vi "Server Main Simplicity.vi"() -> ()   [LabVIEW 2015]
doc: "Use this template to create an application that executes until you click the Stop button. Unlike the Single Loop Application VI that uses polling, this VI uses the Event structure."
uses:
  Type/_Server Command.ctl
  Type/_Run State.ctl
  Type/_Log Command.ctl
  <vilib>/registry/registry.llb/Registry SAM.ctl
  Type/_RT Command.ctl
  Configuration/AcquisitionState.ctl
  Type/_RT Instrument State.ctl
  Type/_Source Type.ctl
  <vilib>/Utility/config.llb/Read Key (Path).vi
  <vilib>/Utility/config.llb/Write Key (Path).vi
  <vilib>/Utility/config.llb/Read Key (String).vi
  <vilib>/Utility/config.llb/Write Key (String).vi
  Configuration/_Global Configuration.vi
  <vilib>/registry/registry.llb/Write Registry Value Simple STR.vi
  <vilib>/Utility/config.llb/Read Key (Boolean).vi
  <vilib>/Utility/config.llb/Read Key (I32).vi
  _Server Global.vi
  <vilib>/Utility/config.llb/NI_LVConfig.lvlib
panel:
  out "MS Status":string="Simulation (State = Ready)"
  in  "MSStatusWindow":bool
  in  "MSShutDown":bool
  in  "MSStart":bool
  out "S2Type":i8(ring)=2 items=["None", "ESI", "APCI", "APPI", "MicroSpray"]
  out "S1Type":i8(ring)=1 items=["None", "ESI", "APCI", "APPI", "MicroSpray"]
  out "S2Temp":sgl caption="Data Queue"
  out "S1Temp":sgl=125.0 caption="Data Queue"
  out "HSIDTemp":sgl=300.0 caption="Data Queue"
  in  "Negative":bool
  in  "Positive":bool
  out "MS Ready":u16(ring)=2
  in  "ContactClosures":bool
  out "Corona Discharge:":sgl format="%.1f"
  out "ElectroSpray V2:":sgl
  out "ElectroSpray V1:":sgl
  in  "GetStatus":bool
  out "Heating Gas 2:":sgl
  out "Heating Gas 1:":sgl
  out "Nebulizer Gas 1:":sgl
  out "Nebulizer Gas 2:":sgl
  out "Collision Pressure:":sgl format="%.1f"
  out "Dry Gas:":sgl
  out "Exhaust:":sgl
  out "Pump Speed:":sgl
  out "Exhaust OK":bool
  out "CurGas OK":bool
  out "Pump OK":bool
  out "Interlock OK":bool
  out "Vac. Pressure:":sgl format="%.2e"
  out "Scans":i32 caption="Data Queue"
  out "Engine Error":errorcluster
  out "Connected":bool
  out "Error":string
  out "Data":string
  out "Ready":bool=TRUE
  in  "Command":T1=enum."Get Status"
  in  "Message":string="<Method>\n  1\t0\t0\n  <Experiment>\n    1\t0\t0\t200\t0\t100\t1\t0\n    <MassRange>\n      200.000000\t400\t0.100000\t2000\t0.1\t0\n      <ParamTable/>\n    </MassRange>\n  </Experiment>\n</Method>"
  out "Data Queue":i32
  out "Busy":bool
  out "Locked":bool
  # "Mass Calibration & Resolution"
  # "Source"
  # "1"
  # "2"
  # "HSID"
  # "Simplicity Server V6.5 R&D"
  # "Source 1"
  # "Common Interface"
  # "Source 2"
  # "Other Status"
  # "Torr"
  # "Interlocks:"
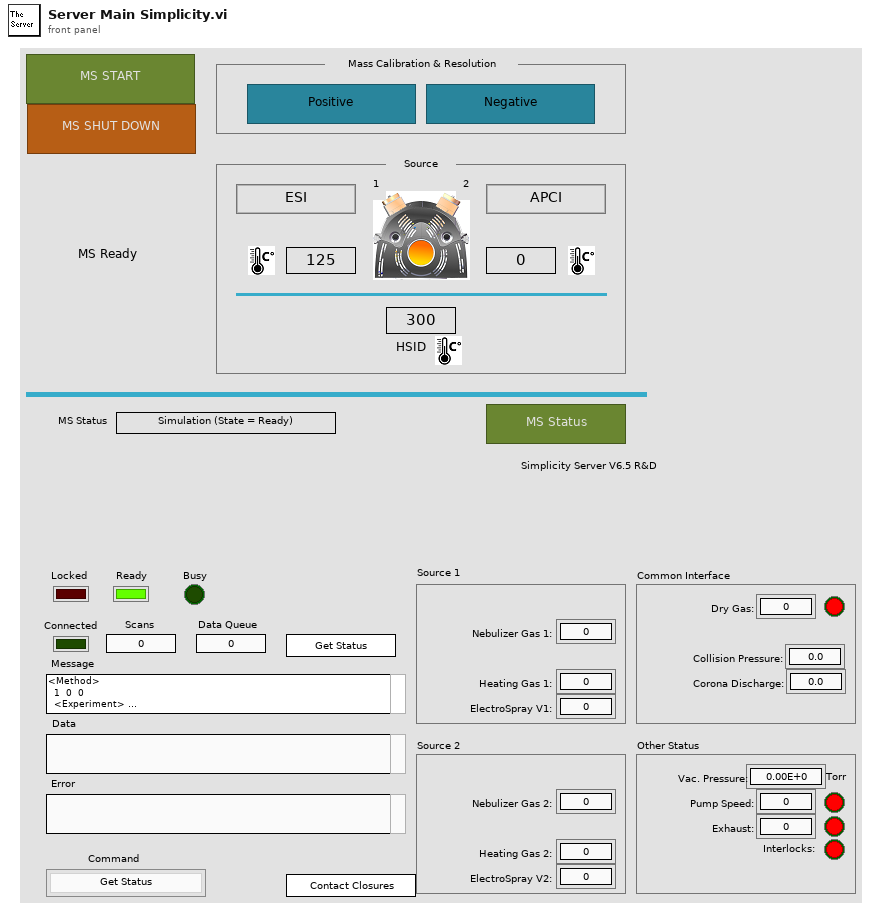
[diagram p1: front panel]
types:
  T1 = typedef "_Server Command.ctl" = enum16{"Hide Server", "Show Server", "Close Server", "Start Run", "Start Actual Run", "Stop Run", "Runtime Update", "Get Data", "Get Status", "Get Table", "Set Table", "Get Configuration", "Reserved", "Get Memory Map", "Read ADC", "Set Oscillator", "Reboot", "Backup Firmware", "Update Firmware", "Auxiliary Update", "System Status", "Start System", "Shutdown System", "Start LC Equilibration", "Get LC Status", "Get LC Configuration", "Get LC Method Contents", "Rinse Autosampler", "Pump OnOff", "Oven OnOff", "Get LC Error", "Clear LC Error", "Set LC Input Logic", "Set LC Hold Logic", "Lock Server", "Get Current Method", "Get Real Time Data", "Connect LC", "Disconnect LC"}
  T2 = typedef "_Run State.ctl" = enum16{"Init", "Update", "Start", "End", "Error"}
  T3 = typedef "_Log Command.ctl" = enum16{"No Command", "Open", "Read", "Write", "Close", "Check Size"}
  T4 = typedef "AcquisitionState.ctl" = enum16{"Ready", "Busy", "Waiting"}
  T5 = enum32{"Invalid", "Standard", "Closed", "Hidden", "Minimized", "Maximized"}
  T6 = typedef "_RT Command.ctl" = enum16{"xml Start Run", "xml Start Actual Run", "xml Stop Run", "xml Runtime Update", "xml Get Status", "xml Get Table", "xml Set Table", "xml Get Configuration", "xml System Status", "xml Set LC Input Logic", "xml Get Data", "xml Get Info", "Start", "StartActualRun", "Stop", "Runtime Update", "Get Data", "Get Info", "Get Status", "Get Param", "Get Config", "Get Table", "Read ADC", "Set Oscillator", "Update Config", "Update Table", "Set All Pol", "Set Pol and DC", "Set Max Mass", "Toggle RP", "Toggle EL", "Set PIC", "Initialize Turbo", "Send Turbo Comm", "Close Turbo", "P1", "P2", "P3", "Send Serial", "Set LC Out", "Get LC In", "Read VAC", "Test Table", "Toggle Power", "Get Startup", "Set Startup", "Get ADC Table", "Set ADC Table", "Get Brief Status", "Get Detail Status", "Auxiliary Update", "Set CC Logics", "Set CC Input Logics", "Ignore Error", "invalid"}
  T7 = typedef "Registry SAM.ctl" = enum32{"KEY_QUERY_VALUE", "KEY_SET_VALUE", "KEY_CREATE_SUB_KEY", "KEY_ENUMERATE_SUB_KEYS", "KEY_NOTIFY", "KEY_CREATE_LINK", "KEY_READ", "KEY_WRITE", "KEY_ALL_ACCESS", "KEY_READ | KEY_WRITE"}
  T8 = enum8{"Enabled", "Disabled", "Disabled and Grayed Out"}
  T9 = enum32{"Bad", "Idle", "Run top level", "Running"}
  T10 = typedef "NI_LVConfig.lvlib/Config Data RefNum.ctl" = refnum<k1>
  T11 = typedef "Registry refnum.ctl" = refnum<k1>
  T12 = typedef "_RT Instrument State.ctl" = enum16{"Initializing", "Mass Spectrometer is Off", "Starting Up", "Turning Power Off", "Going to Standby", "Roughing Pump Ready", "Turning Turbo Off", "Turbo Startup", "Turbopump Ready", "Checking Vacuum", "Going to Ready", "Ready", "Running", "Source Standby", "Lost Communication", "Shutting Down", "Fault", "24V Standby", "Go to 24V Standby", "Turbopump Ready-Waiting"}
  T13 = cluster{"InstrState":T12, "RT Ready":bool, "LockServer":bool, "LastGetStatusTime":u32}
  T14 = typedef "_XML Lens.ctl" = cluster{"Value":dbl, "ChID":u8}
  T15 = typedef "_RT Instrument 2.ctl" = cluster{"Table":T16[], "Instrument":string[]}
  T16 = typedef "_RT Configuration 2.ctl" = cluster{"Name":string, "Ch#":u8, "Min":dbl, "Max":dbl, "Def+":dbl, "Def-":dbl, "Offset":dbl, "Slope":dbl, "Type":u8, "Description":string, "SettleT":dbl}
  T17 = cluster{"value":string, string, path, "Source":enum32{"RT Target", "Folder"}}
  T18 = typedef "_Source Type.ctl" = i8
  T19 = typedef "_Brief Status.ctl" = cluster{"Source 1 Type: ":T18, "Nebulizer Gas 1:":sgl, "Probe Temp 1: ":sgl, "Heating Gas 1:":sgl, "Source 2 Type:  ":T18, "Nebulizer Gas 2:":sgl, "Probe Temp 2: ":sgl, "Heating Gas 2:":sgl, "Dry Gas:":sgl, "HSID Temp:  ":sgl, "Collision Gas:":sgl, "Vac. Pressure: ":sgl, "Pump Speed:":sgl, "Exhaust:":sgl, "Interlock OK":bool, "CurGas OK":bool, "Pump OK":bool, "Exhaust OK":bool, "Event":string, "Corona Discharge:":sgl, "Source 1 Voltage:":sgl, "Source 2 Voltage:":sgl}
  T20 = enum16{"Left Button", "Center Button", "Right Button", "Window Close"}
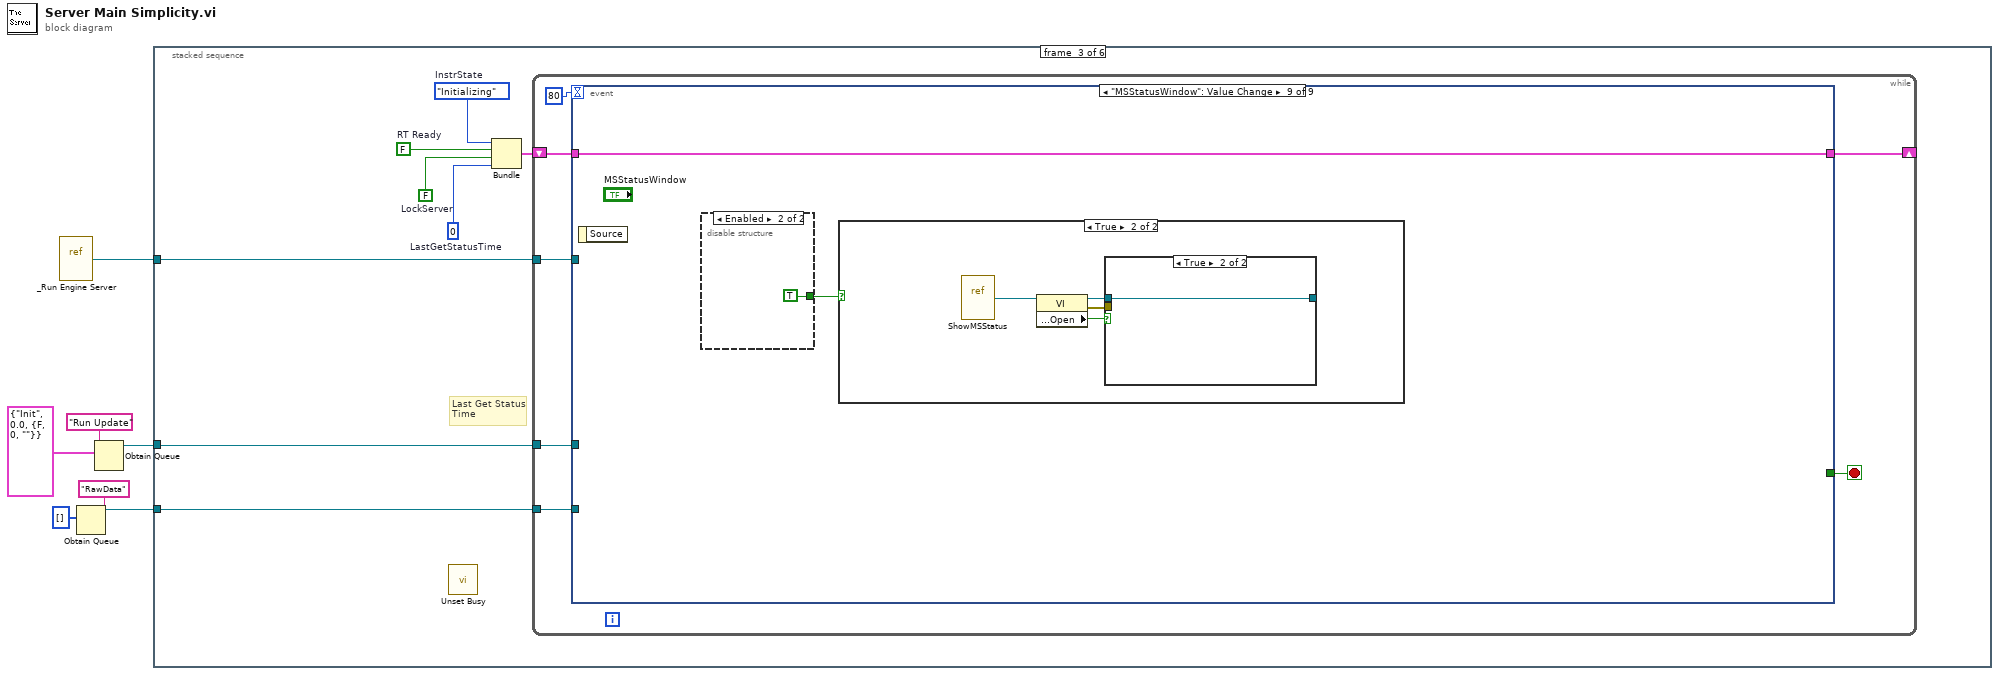
[diagram p0: block diagram]
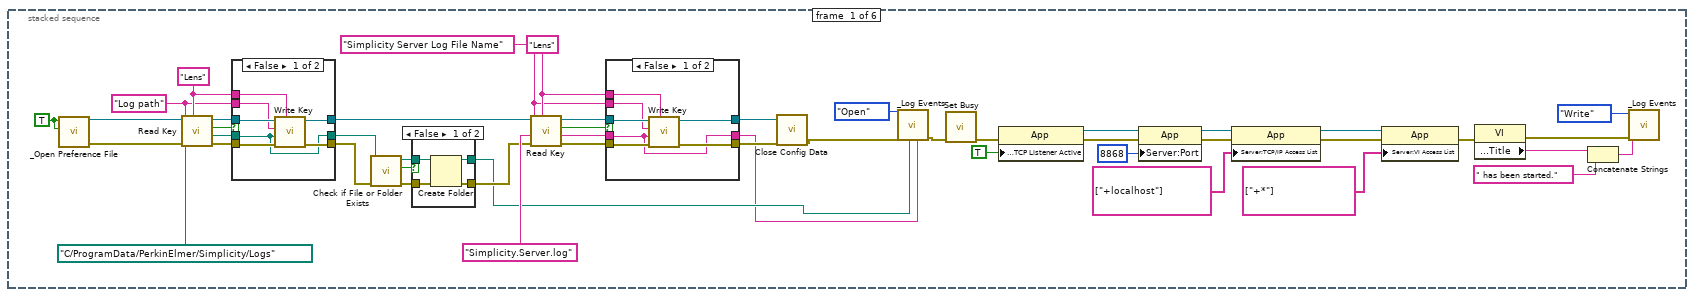
[diagram p2: hidden frame]
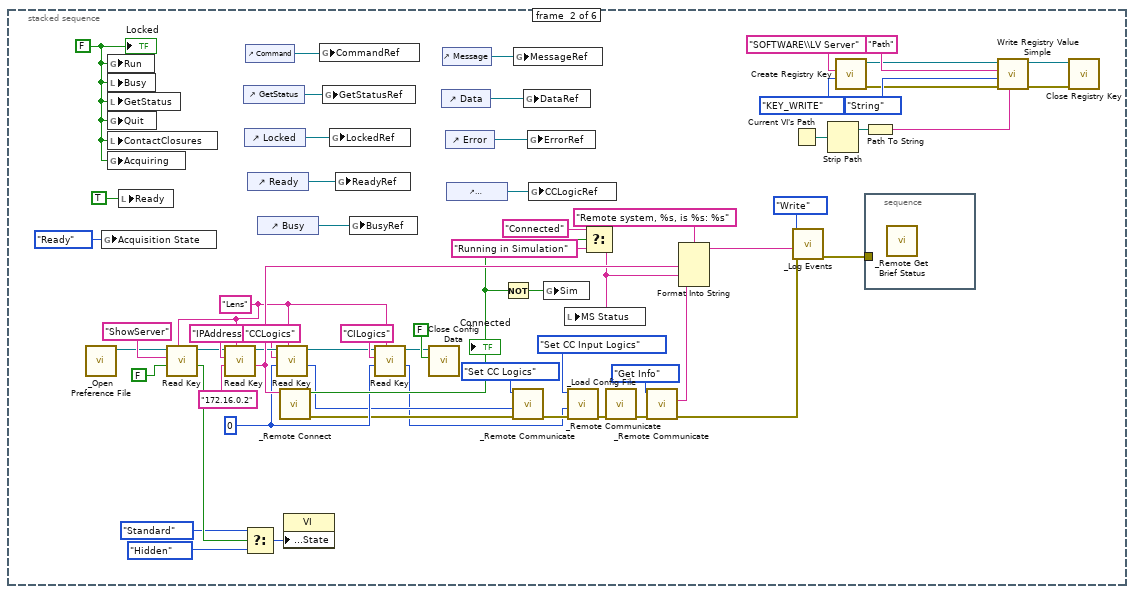
[diagram p6: hidden frame]
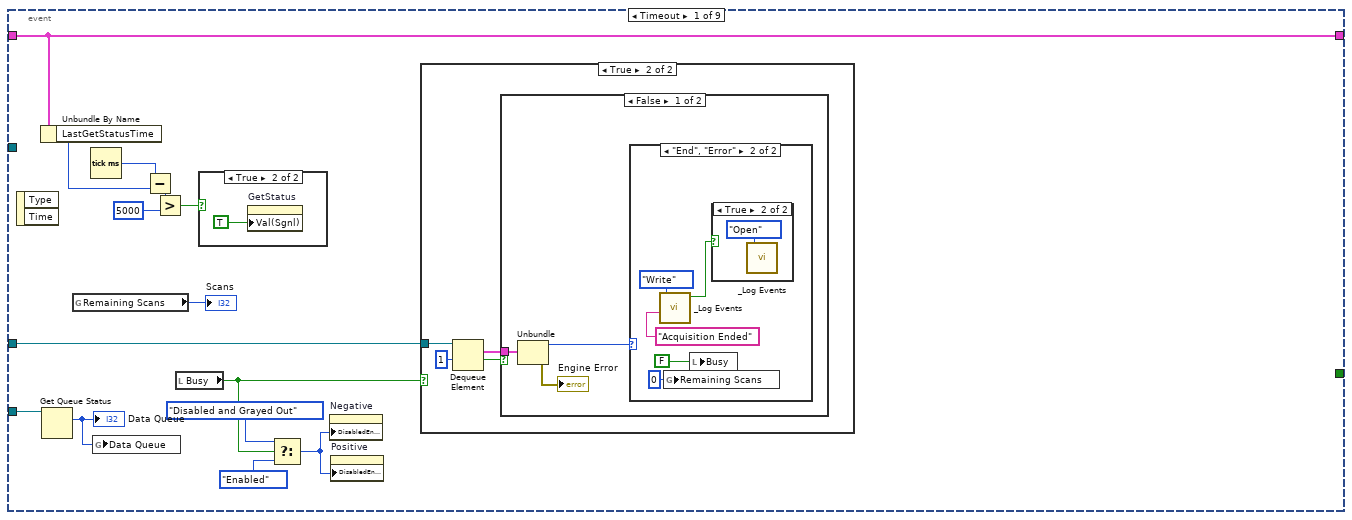
[diagram p7: hidden frame]
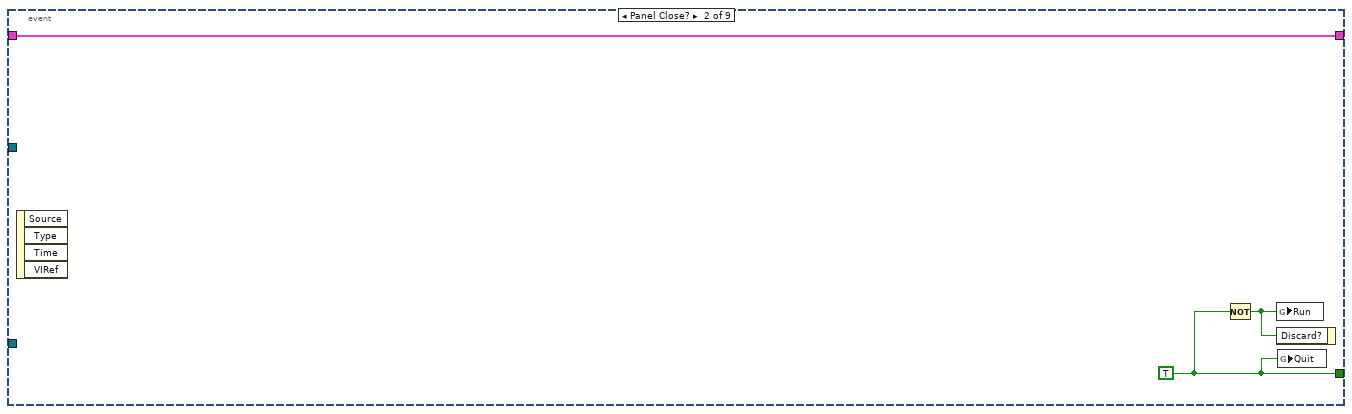
[diagram p13: hidden frame]
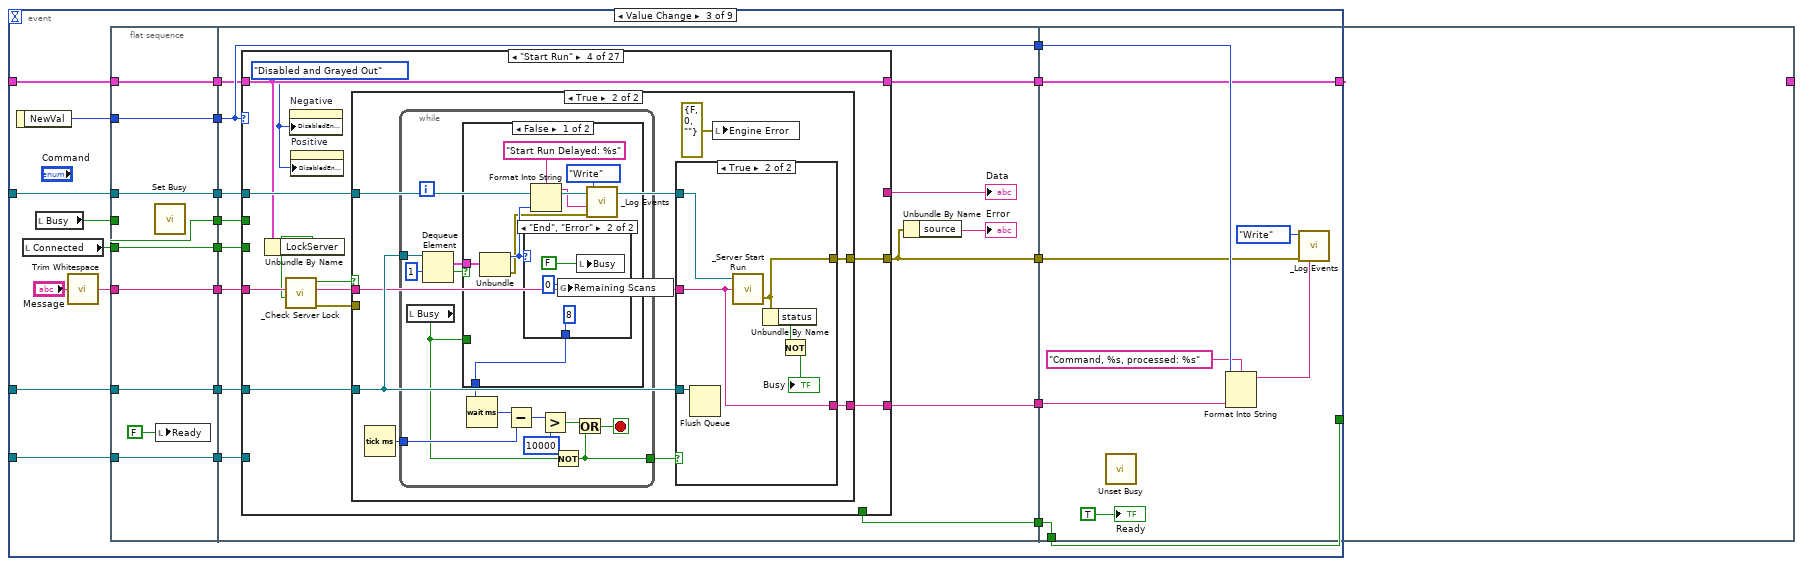
[diagram p14: hidden frame]
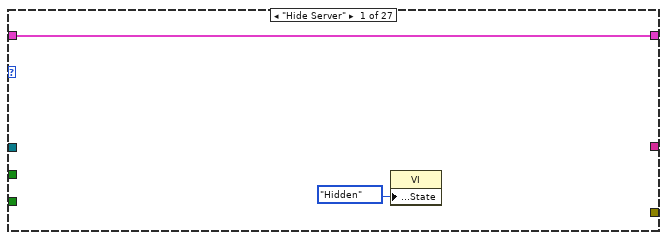
[diagram p15: hidden frame]
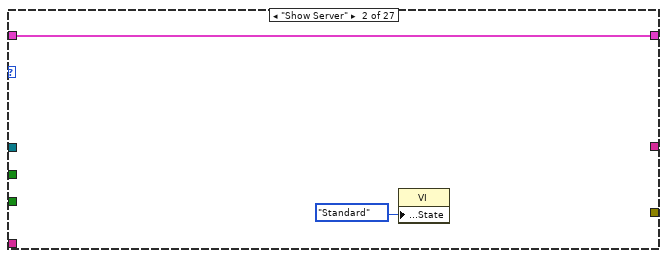
[diagram p16: hidden frame]
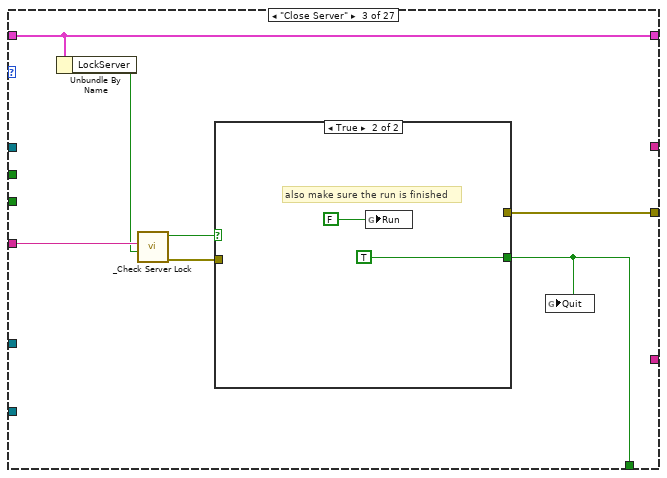
[diagram p17: hidden frame]
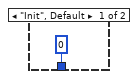
[diagram p20: hidden frame]
diagram:
  n1 = vi-ref "_Run Engine Server.vi"() -> (w5:refnum<vi>)
  n2 = Obtain Queue(name (unnamed)="RawData", element data type=i32[] []) -> (queue out=w1:refnum<queue>)  [unwired: 3 in, 2 out]
  n3 = Obtain Queue(name (unnamed)="Run Update", element data type=cluster{T2, dbl, "error out":errorcluster} {enum."Init", 0.0, "error out"={"status"=FALSE, "code"=0, "source"=""}}) -> (queue out=w4:refnum<queue>)  [unwired: 3 in, 2 out]
  n4 = stacked-sequence {
    tunnel: w4 -> [_ _ w151 _ _ _]
    tunnel: w5 -> [_ _ w150 _ _ _]
    tunnel: w1 -> [_ _ w144 _ _ _]
    frame #0 {
      w21 = "Simplicity Server Log File Name" ("key")
      w22 = "Lens" ("section")
      w27 = "Log path" ("key")
      w28 = "Lens" ("section")
      w36 = TRUE ("Server")
      n5 = call "_Open Preference File.vi"("Initialize"=w36, "Server"=w36) -> ("error"=w17:errorcluster, "refnum"=w18:T10)  [unwired: 1 in, 3 out]
      n6 = call-poly <vilib>:"Read Key.vi"("section"=w28, "error in (no error)"=w17, "default value"=path "C:/ProgramData/PerkinElmer/Simplicity/Logs", "key"=w27, "refnum"=w18) -> ("error out"=w33:errorcluster, "value"=w31:path, "found?"=w32:bool, "refnum out"=w30:T10)  [unwired: 3 in]
      n7 = case shown="False" w32 {
        tunnel: w33 -> [w78 w81]
        tunnel: w31 -> [w72 w79]
        tunnel: w30 -> [w76 w80]
        tunnel: [w77 w81] -> w11
        tunnel: [w75 w80] -> w29
        tunnel: [w72 w79] -> w12
        tunnel: w28 -> [w74 _]
        tunnel: w27 -> [w73 _]
        frame False {
          n8 = call-poly <vilib>:"Write Key.vi"("section"=w74, "error in (no error)"=w78, "value"=w72, "key"=w73, "refnum"=w76) -> ("error out"=w77:errorcluster, "refnum out"=w75:T10)  [unwired: 4 in, 1 out]
        }
        frame True {
        }
      }
      n9 = call <vilib>:"Check if File or Folder Exists.vi"("error in (no error)"=w11, "path"=w12) -> ("error out"=w15:errorcluster, "file or folder exists?"=w13:bool, "dup path"=w14:path)  [unwired: 7 in]
      n10 = case shown="False" w13 {
        tunnel: w15 -> [w59 w60]
        tunnel: w14 -> [w58 w61]
        tunnel: [w57 w61] -> w9
        tunnel: [w56 w60] -> w10
        frame False {
          n11 = Create Folder(path (use dialog)=w58, error in=w59) -> (created path=w57:path, error out=w56:errorcluster)  [unwired: 1 in, 1 out]
        }
        frame True {
        }
      }
      n12 = call-poly <vilib>:"Read Key.vi"("section"=w22, "error in (no error)"=w10, "default value"="Simplicity.Server.log", "key"=w21, "refnum"=w29) -> ("error out"=w23:errorcluster, "value"=w24:string, "found?"=w25:bool, "refnum out"=w26:T10)  [unwired: 3 in]
      n13 = case shown="False" w25 {
        tunnel: w23 -> [w68 w71]
        tunnel: w24 -> [w62 w69]
        tunnel: w26 -> [w66 w70]
        tunnel: [w67 w71] -> w19
        tunnel: [w65 w70] -> w20
        tunnel: [w62 w69] -> w8
        tunnel: w22 -> [w64 _]
        tunnel: w21 -> [w63 _]
        frame False {
          n14 = call-poly <vilib>:"Write Key.vi"("section"=w64, "error in (no error)"=w68, "value"=w62, "key"=w63, "refnum"=w66) -> ("error out"=w67:errorcluster, "refnum out"=w65:T10)  [unwired: 4 in, 1 out]
        }
        frame True {
        }
      }
      n15 = call <vilib>:"Close Config Data.vi"("error in (no error)"=w19, "refnum"=w20) -> ("error out"=w16:errorcluster)  [unwired: 1 in, 8 out]
      n16 = call "_Log Events.vi"("File Name"=w8, "Log Path"=w9, "error in (no error)"=w16, "Log Command"=_Log_Command."Open" ("File Command")) -> ("error out"=w37:errorcluster)  [unwired: 4 in, 1 out]
      n17 = call <vilib>:"Set Busy.vi"("error in (no error)"=w37) -> ("error out"=w39:errorcluster)  [unwired: 3 in, 7 out]
      n18 = property class="App"(error in=w39, "Server:TCP Listener Active"=TRUE) -> (reference out=w54:refnum<vi>, error out=w53:errorcluster)  [unwired: 1 in]
      n19 = property class="App"(reference=w54, error in=w53, "Server:Port"=u32 8868) -> (reference out=w51:refnum<vi>, error out=w50:errorcluster)
      n20 = property class="App"(reference=w51, error in=w50, "Server:TCP/IP Access List"=string[] ["+localhost"]) -> (reference out=w49:refnum<vi>, error out=w48:errorcluster)
      n21 = property class="App"(reference=w49, error in=w48, "Server:VI Access List"=string[] ["+*"]) -> (error out=w41:errorcluster)  [unwired: 1 out]
      n22 = property class="VI"(error in=w41) -> (error out=w40:errorcluster, "Front Panel Window:Title"=w44:string)  [unwired: 1 in, 1 out]
      n23 = Concatenate Strings(w44, " has been started." ("string")) -> (w42:string)
      n24 = call "_Log Events.vi"("error in (no error)"=w40, "Event"=w42, "Log Command"=_Log_Command."Write" ("File Command")) -> ()  [unwired: 5 in, 2 out]
    }
    frame #1 {
      w114 = 0
      w91 = "Lens" ("section")
      w84 = FALSE ("Locked")
      n25 = call "_Open Preference File.vi"() -> ("refnum"=w93:T10)  [unwired: 3 in, 4 out]
      n26 = global write "_Global Configuration.vi" "Acquisition State"(AcquisitionState."Ready" ("Acquisition State")) -> ()
      n27 = global write "_Global Configuration.vi" "Run"(w84) -> ()
      n28 = local write "Busy"(w84) -> ()
      n29 = local write "GetStatus"(w84) -> ()
      n30 = global write "_Global Configuration.vi" "Quit"(w84) -> ()
      n31 = local write "ContactClosures"(w84) -> ()
      n32 = global write "_Global Configuration.vi" "Acquiring"(w84) -> ()
      n33 = local write "Ready"(TRUE ("Ready")) -> ()
      n34 = call-poly <vilib>:"Read Key.vi"("section"=w91, "default value"=FALSE, "key"="ShowServer" ("section"), "refnum"=w93) -> ("value"=w88:bool, "refnum out"=w92:T10)  [unwired: 1 in, 5 out]
      n35 = call-poly <vilib>:"Read Key.vi"("section"=w91, "default value"="172.16.0.2", "key"="IPAddress" ("section"), "refnum"=w92) -> ("value"=w124:string, "refnum out"=w118:T10)  [unwired: 2 in, 4 out]
      n36 = control-ref of="GetStatus"() -> (w104:refnum<vi>)
      n37 = control-ref of="Locked"() -> (w103:refnum<vi>)
      n38 = Select(t=T5."Standard" ("Front Panel Window:State"), s=w88, f=T5."Hidden" ("Front Panel Window:State")) -> (s? t:f=w89:T5)
      n39 = control-ref of="Command"() -> (w105:refnum<vi>)
      n40 = control-ref of="Ready"() -> (w99:refnum<vi>)
      n41 = control-ref of="Busy"() -> (w98:refnum<vi>)
      n42 = call-poly <vilib>:"Read Key.vi"("section"=w91, "default value"=w114, "key"="CCLogics" ("section"), "refnum"=w118) -> ("value"=w109:i32, "refnum out"=w82:T10)  [unwired: 1 in, 5 out]
      n43 = call "_Remote Connect.vi"("IP Address"=w124) -> ("error out"=w108:errorcluster, "TCP"=w119:bool)  [unwired: 1 in, 4 out]
      "Connected" <- w119
      n44 = property class="VI"("Front Panel Window:State"=w89) -> ()  [unwired: 2 in, 2 out]
      n45 = global write "_Server Global.vi" "CommandRef"(w105) -> ()
      n46 = global write "_Server Global.vi" "GetStatusRef"(w104) -> ()
      n47 = global write "_Server Global.vi" "LockedRef"(w103) -> ()
      n48 = global write "_Server Global.vi" "ReadyRef"(w99) -> ()
      n49 = global write "_Server Global.vi" "BusyRef"(w98) -> ()
      n50 = call-poly <vilib>:"Read Key.vi"("section"=w91, "default value"=w114, "key"="CILogics" ("section"), "refnum"=w82) -> ("value"=w107:i32, "refnum out"=w116:T10)  [unwired: 1 in, 5 out]
      n51 = call <vilib>:"Close Config Data.vi"("write file if changed (T)"=FALSE ("write configuration file? (T)"), "refnum"=w116) -> ()  [unwired: 1 in, 9 out]
      n52 = control-ref of="Data"() -> (w101:refnum<vi>)
      n53 = control-ref of="Message"() -> (w102:refnum<vi>)
      n54 = control-ref of="Error"() -> (w100:refnum<vi>)
      n55 = control-ref of="ContactClosures"() -> (w96:refnum<vi>)
      n56 = Not(x=w119) -> (.not. x?=w120:bool)
      n57 = call "_Remote Communicate.vi"("error in (no error)"=w108, "DC Param"=w109, "Command"=_RT_Command."Set CC Logics") -> ("error out"=w110:errorcluster)  [unwired: 3 in, 3 out]
      n58 = global write "_Server Global.vi" "MessageRef"(w102) -> ()
      n59 = global write "_Server Global.vi" "DataRef"(w101) -> ()
      n60 = global write "_Server Global.vi" "ErrorRef"(w100) -> ()
      n61 = global write "_Server Global.vi" "CCLogicRef"(w96) -> ()
      n62 = global write "_Global Configuration.vi" "Sim"(w120) -> ()
      n63 = call "_Remote Communicate.vi"("error in (no error)"=w110, "DC Param"=w107, "Command"=_RT_Command."Set CC Input Logics") -> ("error out"=w112:errorcluster)  [unwired: 3 in, 3 out]
      n64 = Select(t="Connected", s=w119, f="Running in Simulation") -> (s? t:f=w95:string)
      n65 = local write "MS Status"(w95) -> ()
      n66 = call "_Load Config File.vi"("error in (no error)"=w112) -> ("error out"=w121:errorcluster)  [unwired: 6 out]
      n67 = call "_Remote Communicate.vi"("error in (no error)"=w121, "Command"=_RT_Command."Get Info") -> ("error out"=w106:errorcluster, "Info"=w122:string)  [unwired: 4 in, 2 out]
      n68 = Format Into String(format string="Remote system, %s, is %s: %s", w124, w95, w122) -> (resulting string=w128:string)  [unwired: 2 in, 1 out]
      n69 = Current VI's Path() -> (path=w138:path)
      n70 = call "_Log Events.vi"("error in (no error)"=w106, "Event"=w128, "Log Command"=_Log_Command."Write" ("File Command")) -> ("error out"=w97:errorcluster)  [unwired: 5 in, 1 out]
      n71 = Strip Path(path=w138) -> (stripped path=w139:path)  [unwired: 1 out]
      n72 = call <vilib>:"Create Registry Key.vi"("security access mask (KEY_READ | KEY_WRITE)"=Registry_SAM."KEY_WRITE", "subkey"="SOFTWARE\\LV Server") -> ("error out"=w136:errorcluster, "refnum out"=w135:T11)  [unwired: 2 in, 6 out]
      n73 = Path To String(path=w139) -> (string=w140:string)
      n74 = stacked-sequence {
        tunnel: w97 -> [_]
        frame #0 {
          n75 = call "_Remote Get Brief Status.vi"() -> ()  [unwired: 2 in, 3 out]
        }
      }
      n76 = call-poly <vilib>:"Write Registry Value Simple.vi"("String/Binary data"=w140, "error in (no error)"=w136, "simple data type"=enum16{"String", "Binary", "DWORD"}."String", "value"="Path", "refnum"=w135) -> ("error out"=w141:errorcluster, "refnum out"=w142:T11)  [unwired: 3 out]
      n77 = call <vilib>:"Close Registry Key.vi"("error in (no error)"=w141, "refnum"=w142) -> ()  [unwired: 6 out]
      "Locked" <- w84
    }
    frame #2 {
      w145 = _RT_Instrument_State."Initializing"  # InstrState
      w146 = u32 0  # LastGetStatusTime
      w147 = FALSE  # LockServer
      w148 = FALSE  # RT Ready
      # "Last Get Status\nTime"
      n78 = call <vilib>:"Unset Busy.vi"() -> ()  [unwired: 2 in, 10 out]
      n79 = Bundle("InstrState"=w145, "RT Ready"=w148, "LockServer"=w147, "LastGetStatusTime"=w146) -> (w149:T13)  [unwired: 1 out]
      n80 = while {
        tunnel: w151 -> [w156]
        tunnel: w150 -> [w155]
        tunnel: w144 -> [w154]
        shift-right: [w152] -> _
        shift-left: w149 -> [w153]
        stop <- w157 stop-if-true
        n81 = event shown="[8] \"MSStatusWindow\": Value Change" {
          selector: _ -> [_ _ _ _ _ _ _ _ _]
          dyn-events: _ -> [_ _ _ _ _ _ _ _ _]
          timeout: 80 -> [_ _ _ _ _ _ _ _ _]
          tunnel: [_ w187 w211 _ _ _ _ _ _] -> w157
          tunnel: w156 -> [w172 _ w206 _ _ _ _ _ _]
          tunnel: w155 -> [_ _ w207 _ _ _ _ _ _]
          tunnel: w154 -> [w171 _ w205 _ _ _ _ _ _]
          tunnel: w153 -> [w163 w189 w204 w868 w912 w916 w951 w962 w967]
          tunnel: [w163 w189 w203 w881 w912 w916 w951 w962 w967] -> w152
          event Timeout {
            n82 = event-data() -> ()  [unwired: 3 out]
            n83 = Unbundle By Name(w163) -> ("LastGetStatusTime"=w165:u32)
            n84 = Get Queue Status(queue=w171) -> (# elements in queue=w169:i32)  [unwired: 1 in, 8 out]
            "Data Queue" <- w169
            n85 = global read "_Server Global.vi" "Remaining Scans"() -> (→"Scans":i32)
            n86 = Tick Count (ms)() -> (millisecond timer value=w168:u32)
            n87 = global write "_Server Global.vi" "Data Queue"(w169) -> ()
            n88 = Subtract(x=w168, y=w165) -> (x-y=w166:u32)
            n89 = Greater?(x=w166, y=u32 5000) -> (0:w164:bool)
            n90 = local read "Busy"() -> (w162:bool)
            n91 = case shown="True" w164 {
              frame False {
              }
              frame True {
                n92 = property on="GetStatus" class="Bool (strict)"("Val(Sgnl)"=TRUE ("Value (Signaling)")) -> ()  [unwired: 2 in, 2 out]
              }
            }
            n93 = Select(t=T8."Disabled and Grayed Out" ("Disabled"), s=w162, f=T8."Enabled" ("Disabled")) -> (s? t:f=w159:T8)
            n94 = property on="Negative" class="Bool"("DisabledEnum"=w159) -> ()  [unwired: 2 in, 2 out]
            n95 = property on="Positive" class="Bool"("DisabledEnum"=w159) -> ()  [unwired: 2 in, 2 out]
            n96 = case shown="True" w162 {
              tunnel: w172 -> [_ w176]
              frame False {
              }
              frame True {
                n97 = Dequeue Element(queue=w176, timeout in ms (-1)=1) -> (element=w174:cluster{T2, dbl, "error out":errorcluster}, timed out?=w175:bool)  [unwired: 1 in, 2 out]
                n98 = case shown="False" w175 {
                  tunnel: w174 -> [w180 _]
                  frame False {
                    n99 = Unbundle(w180) -> (w178:T2, "error out"=→"Engine Error":errorcluster)  [unwired: 1 out]
                    n100 = case shown="\"End\", \"Error\"" w178 {
                      frame "Init", Default {
                      }
                      frame "End", "Error" {
                        n101 = call "_Log Events.vi"("Event"="Acquisition Ended", "Log Command"=_Log_Command."Write" ("File Command")) -> (">10MB"=w181:bool)  [unwired: 6 in, 1 out]
                        n102 = global write "_Server Global.vi" "Remaining Scans"(0 ("Remaining Scans")) -> ()
                        n103 = local write "Busy"(FALSE ("Running")) -> ()
                        n104 = case shown="True" w181 {
                          frame False {
                          }
                          frame True {
                            n105 = call "_Log Events.vi"("Log Command"=_Log_Command."Open" ("File Command")) -> ()  [unwired: 7 in, 2 out]
                          }
                        }
                      }
                    }
                  }
                  frame True {
                  }
                }
              }
            }
          }
          event Panel Close? {
            w187 = TRUE ("RT Ready")
            n106 = event-data() -> ()  [unwired: 5 out]
            n107 = Not(x=w187) -> (.not. x?=w188:bool)
            n108 = global write "_Global Configuration.vi" "Run"(w188) -> ()
            n109 = event-data("Discard?"=w188) -> ()  [unwired: 1 in, 1 out]
            n110 = global write "_Global Configuration.vi" "Quit"(w187) -> ()
          }
          event Value Change {
            n111 = event-data() -> ("NewVal"=w213:T1)  [unwired: 1 out]
            n112 = local read "Connected"() -> (w208:bool)
            n113 = local read "Busy"() -> (w210:bool)
            n114 = call <vilib>:"Trim Whitespace.vi"("string"="Message") -> ("trimmed string"=w209:string)  [unwired: 1 in]
            n115 = flat-sequence {
              tunnel: w213 -> [w221]
              tunnel: [w221] -> w202
              tunnel: w209 -> [w220]
              tunnel: [w220] -> w201
              tunnel: w210 -> [w219]
              tunnel: [w219] -> w200
              tunnel: w208 -> [w218]
              tunnel: [w218] -> w199
              tunnel: w207 -> [w217]
              tunnel: [w217] -> w198
              tunnel: w206 -> [w216]
              tunnel: [w216] -> w197
              tunnel: w205 -> [w215]
              tunnel: [w215] -> w196
              tunnel: w204 -> [w214]
              tunnel: [w214] -> w195
              tunnel: w202 -> [w236]
              tunnel: [w236] -> w194
              tunnel: w201 -> [w234]
              tunnel: [w233] -> w193
              tunnel: w200 -> [w231]
              tunnel: w199 -> [w230]
              tunnel: w198 -> [w223]
              tunnel: w197 -> [w228]
              tunnel: w196 -> [w227]
              tunnel: w195 -> [w225]
              tunnel: [w224] -> w192
              tunnel: [w229] -> w191
              tunnel: [w226] -> w190
              tunnel: w194 -> [w860]
              tunnel: [w854] -> w211
              tunnel: w193 -> [w854]
              tunnel: [w853] -> w203
              tunnel: w192 -> [w853]
              tunnel: w191 -> [w857]
              tunnel: w190 -> [w855]
              frame #0 {
                n116 = call <vilib>:"Set Busy.vi"() -> ()  [unwired: 10 in, 2 out]
                n117 = local write "Ready"(FALSE ("Ready")) -> ()
              }
              frame #1 {
                n118 = case shown="\"Start Run\"" w236 {
                  selector: w236 -> [_ _ _ _ _ _ _ _ _ _ _ _ _ _ _ _ _ _ _ _ _ _ _ _ _ _ w852]
                  tunnel: [_ _ _ _ _ _ _ w395 w455 w466 _ w542 _ w566 w583 _ _ _ _ w757 w774 _ _ w806 w821 _ _] -> w235
                  tunnel: w234 -> [_ _ w247 w258 _ w329 w357 w392 _ w464 w515 _ _ _ _ w601 w627 w651 w702 w756 _ w787 w798 w810 w819 w838 _]
                  tunnel: [_ _ w241 _ _ _ _ _ _ _ _ _ _ _ _ _ _ _ _ _ _ _ _ _ _ _ _] -> w233
                  tunnel: [_ _ w245 w262 w312 w330 w359 w393 w460 w463 w516 w543 _ w576 w594 w603 _ w653 w704 w758 w777 w788 w799 w807 w822 w834 w848] -> w229
                  tunnel: w231 -> [_ _ _ _ _ _ w358 _ _ _ _ _ _ _ _ w602 _ w654 w705 _ _ _ _ _ _ w836 _]
                  tunnel: w230 -> [_ _ _ _ _ _ _ _ _ w467 _ w551 _ _ _ _ w629 w652 w703 _ _ _ _ _ _ _ _]
                  tunnel: w223 -> [_ _ _ w261 w311 w331 _ _ _ _ _ _ _ _ _ _ _ _ _ _ _ _ _ _ _ _ _]
                  tunnel: w228 -> [_ _ _ w259 _ _ _ _ _ _ _ _ _ _ _ _ _ _ _ _ _ _ _ _ _ _ _]
                  tunnel: w227 -> [_ _ _ _ _ _ _ w396 _ _ _ _ _ _ _ _ _ _ _ _ _ _ _ _ _ _ _]
                  tunnel: [_ _ _ w260 _ _ w356 w394 w452 w464 w514 _ _ w566 _ w600 w628 w650 w701 w755 _ _ _ _ _ _ _] -> w226
                  tunnel: w225 -> [w237 w239 w242 w253 w316 w326 w353 w387 w454 w462 w511 w540 w565 w570 w577 w597 w625 w647 w698 w752 w768 w784 w795 w805 w820 w832 w846]
                  tunnel: [w237 w239 w242 w253 w316 w326 w353 w386 w454 w462 w511 w540 w565 w570 w577 w597 w625 w647 w698 w752 w768 w784 w795 w805 w820 w831 w846] -> w224
                  frame "Hide Server" {
                    n119 = property class="VI"("Front Panel Window:State"=T5."Hidden") -> ()  [unwired: 2 in, 2 out]
                  }
                  frame "Show Server" {
                    n120 = property class="VI"("Front Panel Window:State"=T5."Standard") -> ()  [unwired: 2 in, 2 out]
                  }
                  frame "Close Server" {
                    n121 = Unbundle By Name(w242) -> ("LockServer"=w243:bool)
                    n122 = call "_Check Server Lock.vi"("LockServer"=w243, "Message In"=w247) -> ("error out"=w244:errorcluster, "Proceed"=w246:bool)  [unwired: 4 out]
                    n123 = case shown="True" w246 {
                      selector: w246 -> [w249 _]
                      tunnel: [w249 TRUE] -> w241
                      tunnel: [w248 _] -> w245
                      tunnel: w244 -> [w248 _]
                      frame False {
                      }
                      frame True {
                        # "also make sure the run is finished"
                        n124 = global write "_Global Configuration.vi" "Run"(FALSE ("Running")) -> ()
                      }
                    }
                    n125 = global write "_Global Configuration.vi" "Quit"(w241) -> ()
                  }
                  frame "Start Run" {
                    w252 = T8."Disabled and Grayed Out" ("Disabled")
                    n126 = Unbundle By Name(w253) -> ("LockServer"=w254:bool)
                    n127 = call "_Check Server Lock.vi"("LockServer"=w254, "Message In"=w258) -> ("error out"=w255:errorcluster, "Message Out"=w257:string, "Proceed"=w256:bool)  [unwired: 3 out]
                    n128 = property on="Negative" class="Bool"("DisabledEnum"=w252) -> ()  [unwired: 2 in, 2 out]
                    n129 = property on="Positive" class="Bool"("DisabledEnum"=w252) -> ()  [unwired: 2 in, 2 out]
                    n130 = case shown="True" w256 {
                      tunnel: [w263 w272] -> w262
                      tunnel: w261 -> [_ w271]
                      tunnel: [w264 w270] -> w260
                      tunnel: w259 -> [_ w267]
                      tunnel: w257 -> [w264 w265]
                      tunnel: w255 -> [w263 _]
                      frame False {
                      }
                      frame True {
                        n131 = Tick Count (ms)() -> (millisecond timer value=w269:u32)
                        n132 = while {
                          tunnel: w269 -> [w285]
                          tunnel: w267 -> [w277]
                          tunnel: [w276] -> w268
                          stop <- w281 stop-if-true
                          n133 = local read "Busy"() -> (w273:bool)
                          n134 = Dequeue Element(queue=w277, timeout in ms (-1)=1) -> (element=w278:cluster{T2, dbl, "error out":errorcluster}, timed out?=w279:bool)  [unwired: 1 in, 2 out]
                          n135 = case shown="False" w279 {
                            tunnel: w278 -> [w292 _]
                            tunnel: [w286 w297] -> w274
                            tunnel: w273 -> [_ w300]
                            frame False {
                              n136 = Unbundle(w292) -> (w291:T2, "error out"=w287:errorcluster)  [unwired: 1 out]
                              n137 = case shown="\"End\", \"Error\"" w291 {
                                tunnel: [u32 0 ("milliseconds to wait") u32 8 ("milliseconds to wait")] -> w286
                                frame "Init", Default {
                                }
                                frame "End", "Error" {
                                n138 = global write "_Server Global.vi" "Remaining Scans"(0 ("Remaining Scans")) -> ()
                                n139 = local write "Busy"(FALSE ("Running")) -> ()
                                }
                              }
                              n140 = Format Into String(format string="Start Run Delayed: %s", w291) -> (resulting string=w288:string)  [unwired: 2 in, 1 out]
                              n141 = call "_Log Events.vi"("error in (no error)"=w287, "Event"=w288, "Log Command"=_Log_Command."Write" ("File Command")) -> ()  [unwired: 5 in, 2 out]
                            }
                            frame True {
                              n142 = Select(t=u32 38 ("milliseconds to wait"), s=w300, f=u32 0) -> (s? t:f=w297:u32)
                            }
                          }
                          n143 = Wait (ms)(milliseconds to wait=w274) -> (millisecond timer value=w275:u32)
                          n144 = Subtract(x=w275, y=w285) -> (x-y=w284:u32)
                          n145 = Greater?(x=w284, y=u32 10000) -> (0:w282:bool)
                          n146 = Not(x=w273) -> (.not. x?=w276:bool)
                          n147 = Or(x=w282, y=w276) -> (x .or. y?=w281:bool)
                        }
                        n148 = case shown="True" w268 {
                          tunnel: w265 -> [w303 w306]
                          tunnel: [w304 w309] -> w272
                          tunnel: w267 -> [_ w307]
                          tunnel: w271 -> [_ w310]
                          tunnel: [w303 w306] -> w270
                          frame False {
                            n149 = call "_Construct Error Cluster.vi"("reason"="8008: Failed to start a run: 10s timeout while waiting for engine to become ready." ("trimmed string"), "errorCode"=8008) -> ("error out"=w304:errorcluster)  [unwired: 2 in, 3 out]
                          }
                          frame True {
                            n150 = Flush Queue(queue=w307) -> ()  [unwired: 1 in, 3 out]
                            n151 = call "_Server Start Run.vi"("Run Method"=w306, "Eng Refnum"=w310) -> ("error out"=w309:errorcluster)  [unwired: 1 in, 1 out]
                            n152 = Unbundle By Name(w309) -> ("status"=w308:bool)
                            n153 = Not(x=w308) -> (.not. x?=→"Busy":bool)
                          }
                        }
                        n154 = local write "Engine Error"(errorcluster {"status"=FALSE, "code"=0, "source"=""} ("Engine Error")) -> ()
                      }
                    }
                  }
                  frame "Start Actual Run" {
                    n155 = call "_Remote Communicate.vi"("Command"=_RT_Command."StartActualRun") -> ("error out"=w313:errorcluster)  [unwired: 5 in, 3 out]
                    n156 = global read "_Global Configuration.vi" "TCP"() -> (w314:bool)
                    n157 = case shown="False" w314 {
                      tunnel: w311 -> [w321 _]
                      tunnel: [w320 w323] -> w312
                      tunnel: w313 -> [w319 w323]
                      frame False {
                        w322 = FALSE ("Wait until done")
                        n158 = invoke class="VI" method="Run VI"(reference=w321, error in=w319, "Wait until done"=w322, "Auto Dispose Ref"=w322) -> (error out=w320:errorcluster)  [unwired: 1 in, 4 out]
                        n159 = global write "_Global Configuration.vi" "Acquiring"(TRUE ("Acquiring")) -> ()
                        n160 = global write "_Global Configuration.vi" "Run"(TRUE ("Acquiring")) -> ()
                      }
                      frame True {
                      }
                    }
                  }
                  frame "Stop Run" {
                    n161 = Unbundle By Name(w326) -> ("RT Ready"=w324:bool, "LockServer"=w325:bool)
                    n162 = call "_Check Server Lock.vi"("LockServer"=w325, "Message In"=w329) -> ("error out"=w327:errorcluster, "Proceed"=w328:bool)  [unwired: 4 out]
                    n163 = case shown="True" w328 {
                      tunnel: w331 -> [_ w335]
                      tunnel: w324 -> [_ w334]
                      tunnel: [w332 w333] -> w330
                      tunnel: w327 -> [w332 _]
                      frame False {
                      }
                      frame True {
                        n164 = stacked-sequence {
                          tunnel: w335 -> [_ w339 _ _]
                          tunnel: w334 -> [_ _ _ w347]
                          tunnel: [_ _ _ w346] -> w333
                          frame #0 {
                            n165 = global read "_Global Configuration.vi" "TCP"() -> (w336:bool)
                            n166 = case shown="False" w336 {
                              frame False {
                                n167 = global write "_Global Configuration.vi" "Acquisition State"(AcquisitionState."Ready" ("Acquisition State")) -> ()
                              }
                              frame True {
                              }
                            }
                            n168 = global write "_Global Configuration.vi" "Run"(FALSE ("Running")) -> ()
                          }
                          frame #1 {
                            n169 = while {
                              tunnel: w339 -> [w344]
                              stop <- w341 stop-if-true
                              n170 = property class="VI"(reference=w344) -> ("Exec.State"=w343:T9)  [unwired: 1 in, 2 out]
                              n171 = Wait (ms)(milliseconds to wait=u32 180) -> ()  [unwired: 1 out]
                              n172 = Equal?(x=w343, y=T9."Idle") -> (x = y?=w341:bool)
                            }
                          }
                          frame #2 {
                            n173 = Wait (ms)(milliseconds to wait=u32 800) -> ()  [unwired: 1 out]
                          }
                          frame #3 {
                            n174 = case shown="True" w347 {
                              tunnel: [_ w350] -> w346
                              frame False {
                              }
                              frame True {
                                n175 = call "_Remote Wait Until Done.vi"() -> ("error out"=w349:errorcluster)  [unwired: 2 in, 1 out]
                                n176 = call "_Remote Park Lens.vi"("error in"=w349) -> ("error out"=w350:errorcluster)  [unwired: 1 in, 5 out]
                                n177 = global write "_Global Configuration.vi" "Acquiring"(FALSE ("Acquiring")) -> ()
                              }
                            }
                          }
                        }
                      }
                    }
                  }
                  frame "Runtime Update" {
                    n178 = Unbundle By Name(w353) -> ("RT Ready"=w351:bool, "LockServer"=w352:bool)
                    n179 = call "_Check Server Lock.vi"("LockServer"=w352, "Message In"=w357) -> ("error out"=w354:errorcluster, "Message Out"=w356:string, "Proceed"=w355:bool)  [unwired: 3 out]
                    n180 = case shown="True" w355 {
                      tunnel: [w360 w364] -> w359
                      tunnel: w358 -> [_ w363]
                      tunnel: w351 -> [_ w362]
                      tunnel: w356 -> [_ w361]
                      tunnel: w354 -> [w360 _]
                      frame False {
                      }
                      frame True {
                        n181 = case shown="True" w362 {
                          tunnel: w361 -> [_ w367]
                          tunnel: [_ w366] -> w364
                          tunnel: w363 -> [_ w365]
                          frame False {
                          }
                          frame True {
                            n182 = stacked-sequence {
                              tunnel: w367 -> [w372 _]
                              tunnel: [w370 _] -> w366
                              tunnel: w365 -> [w368 _]
                              frame #0 {
                                # "Update a set of lens parameters"
                                n183 = call "_Read XML Lens.vi"("XML String"=w372) -> ("error out"=w371:errorcluster, "Lens"=w369:T14[])  [unwired: 1 in, 4 out]
                                n184 = call "_Server BlockUpdate.vi"("error in"=w371, "Lens"=w369, "Running"=w368) -> ("error out"=w370:errorcluster)  [unwired: 1 in, 3 out]
                              }
                              frame #1 {
                                # "Ensured runtime update has been\napplied at the end of a scan cycle"
                                n185 = Tick Count (ms)() -> (millisecond timer value=w373:u32)
                                n186 = global read "_Server Global.vi" "Remaining Scans"() -> (w374:i32)
                                n187 = while {
                                tunnel: w374 -> [w384]
                                tunnel: w373 -> [w381]
                                stop <- w375 stop-if-true
                                n188 = global read "_Server Global.vi" "Remaining Scans"() -> (w385:i32)
                                n189 = Wait (ms)(milliseconds to wait=u32 80) -> (millisecond timer value=w382:u32)
                                n190 = Equal To 0?(x=w384) -> (x = 0?=w378:bool)
                                n191 = Not Equal?(x=w384, y=w385) -> (x != y?=w377:bool)
                                n192 = Subtract(x=w382, y=w381) -> (x-y=w380:u32)
                                n193 = Greater?(x=w380, y=u32 5000) -> (0:w376:bool)
                                n194 = Compound Arithmetic op=OR(w378, w377, w376) -> (w375:bool)
                                }
                              }
                            }
                          }
                        }
                      }
                    }
                  }
                  frame "Get Data" {
                    n195 = Unbundle By Name(w387) -> ("LockServer"=w388:bool)
                    n196 = call "_Check Server Lock.vi"("LockServer"=w388, "Message In"=w392) -> ("error out"=w389:errorcluster, "Message Out"=w391:string, "Proceed"=w390:bool)  [unwired: 3 out]
                    n197 = case shown="True" w390 {
                      tunnel: w396 -> [_ w409]
                      tunnel: [_ w400] -> w395
                      tunnel: [w399 w405] -> w394
                      tunnel: [w398 w402] -> w393
                      tunnel: w391 -> [w399 w403]
                      tunnel: w389 -> [w398 _]
                      tunnel: w387 -> [w397 w401]
                      tunnel: [w397 w401] -> w386
                      frame False {
                      }
                      frame True {
                        # "Synchronous GetData call will wait for up to 10s for the next expt data for DDE application"
                        n198 = To Lower Case(string=w403) -> (all lower case string=w406:string)
                        n199 = stacked-sequence {
                          tunnel: [w410 _] -> w402
                          frame #0 {
                            n200 = local read "Engine Error"() -> (w410:errorcluster)
                          }
                          frame #1 {
                            n201 = local write "Engine Error"(errorcluster {"status"=FALSE, "code"=0, "source"=""} ("Engine Error")) -> ()
                          }
                        }
                        n202 = Equal?(x=w406, y="synchronous") -> (x = y?=w407:bool)
                        n203 = case shown="True" w407 {
                          tunnel: w409 -> [w416 w433]
                          tunnel: [w415 w430] -> w400
                          tunnel: [w413 w429] -> w404
                          frame False {
                            n204 = while {
                              tunnel: w416 -> [w423]
                              shift-right: [w422] -> w415
                              shift-left: "" -> [w421]
                              tunnel: [w417] -> w414 mode=indexing
                              stop <- w418 stop-if-true
                              n205 = Dequeue Element(queue=w423, timeout in ms (-1)=0) -> (element=w420:i32[], timed out?=w418:bool)  [unwired: 1 in, 2 out]
                              n206 = case shown="False" w418 {
                                tunnel: w420 -> [w427 _]
                                tunnel: [w426 w428] -> w422
                                tunnel: w421 -> [w425 w428]
                                tunnel: [w424 w428] -> w417
                                frame False {
                                n207 = call "_Write XML Data.vi"("Data (1D-I32)"=w427, "PrevString"=w425) -> ("Header"=w424:string, "XML String"=w426:string)  [unwired: 1 in, 3 out]
                                }
                                frame True {
                                }
                              }
                            }
                            n208 = Index Array(array=w414) -> (element=w413:string)  [unwired: 1 in]
                          }
                          frame True {
                            n209 = Tick Count (ms)() -> (millisecond timer value=w432:u32)
                            n210 = while {
                              tunnel: w433 -> [w446]
                              tunnel: w432 -> [w442]
                              tunnel: [w434] -> w431
                              stop <- w435 stop-if-true
                              n211 = Wait (ms)(milliseconds to wait=u32 1) -> (millisecond timer value=w443:u32)
                              n212 = Dequeue Element(queue=w446, timeout in ms (-1)=0) -> (element=w434:i32[])  [unwired: 1 in, 3 out]
                              n213 = Subtract(x=w443, y=w442) -> (x-y=w441:u32)
                              n214 = Array Size(array=w434) -> (size(s)=w439:i32)
                              n215 = Greater?(x=w441, y=u32 10000) -> (0:w437:bool)
                              n216 = Greater?(x=w439, y=2) -> (0:w436:bool)
                              n217 = Or(x=w437, y=w436) -> (x .or. y?=w435:bool)
                            }
                            n218 = call "_Write XML Data.vi"("Data (1D-I32)"=w431) -> ("Header"=w429:string, "XML String"=w430:string)  [unwired: 1 in, 4 out]
                          }
                        }
                        n219 = Concatenate Strings(w406, w404) -> (w405:string)
                      }
                    }
                  }
                  frame "Get Status" {
                    w456 = "\r\n"
                    n220 = global read "_Global Configuration.vi" "Acquisition State"() -> (w449:T4)
                    n221 = call "_Remote Communicate.vi"("Command"=_RT_Command."Get Status") -> ("error out"=w458:errorcluster, "Info"=w453:string)  [unwired: 5 in, 2 out]
                    n222 = Add(x=w449, y=2) -> (x+y=w448:i32)
                    n223 = call "_Remote Communicate.vi"("error in (no error)"=w458, "Command"=_RT_Command."Get Info") -> ("error out"=w460:errorcluster, "Info"=w457:string)  [unwired: 4 in, 2 out]
                    n224 = Format Into String(format string="%d: Ionica Server is %s", w448, w449) -> (resulting string=w450:string)  [unwired: 2 in, 1 out]
                    n225 = Concatenate Strings(w450, w453) -> (w452:string)
                    n226 = Concatenate Strings(w450, w456, w453, w456, w457) -> (w455:string)
                  }
                  frame "Get Table" {
                    # "Outputs 2 2D-DBL table in XML format\n- 1st column is mass in amu\n- 2nd column is DAC value"
                    n227 = Decimal String To Number(string=w464) -> (number=w465:i32)  [unwired: 3 out]
                    n228 = case shown="True" w467 {
                      tunnel: [_ w504] -> w469
                      tunnel: [w486 w505] -> w468
                      tunnel: w465 -> [w487 w507]
                      frame False {
                        n229 = case shown="0, Default" w487 {
                          tunnel: [w488 w489 w490 w491 w492 w493 w494 w495 w496 w497 w498 w499 w500 w501 w502 w503] -> w486
                          frame 0, Default {
                            n230 = global read "_Global Configuration.vi" "Calibration"() -> (w488:dbl[][])
                          }
                          frame 1 {
                            n231 = global read "_Global Configuration.vi" "Calibration 2"() -> (w489:dbl[][])
                          }
                          frame 2 {
                            n232 = global read "_Global Configuration.vi" "Calibration 3"() -> (w490:dbl[][])
                          }
                          frame 3 {
                            n233 = global read "_Global Configuration.vi" "Calibration 4"() -> (w491:dbl[][])
                          }
                          frame 4 {
                            n234 = global read "_Global Configuration.vi" "Resolution"() -> (w492:dbl[][])
                          }
                          frame 5 {
                            n235 = global read "_Global Configuration.vi" "Resolution 2"() -> (w493:dbl[][])
                          }
                          frame 6 {
                            n236 = global read "_Global Configuration.vi" "Resolution 3"() -> (w494:dbl[][])
                          }
                          frame 7 {
                            n237 = global read "_Global Configuration.vi" "Resolution 4"() -> (w495:dbl[][])
                          }
                          frame 8 {
                            n238 = global read "_Global Configuration.vi" "Resolution 5"() -> (w496:dbl[][])
                          }
                          frame 9 {
                            n239 = global read "_Global Configuration.vi" "Resolution 6"() -> (w497:dbl[][])
                          }
                          frame 10 {
                            n240 = global read "_Global Configuration.vi" "Resolution 7"() -> (w498:dbl[][])
                          }
                          frame 11 {
                            n241 = global read "_Global Configuration.vi" "Resolution 8"() -> (w499:dbl[][])
                          }
                          frame 12 {
                            n242 = global read "_Global Configuration.vi" "Resolution 9"() -> (w500:dbl[][])
                          }
                          frame 13 {
                            n243 = global read "_Global Configuration.vi" "Resolution 10"() -> (w501:dbl[][])
                          }
                          frame 14 {
                            n244 = global read "_Global Configuration.vi" "Resolution 11"() -> (w502:dbl[][])
                          }
                          frame 15 {
                            n245 = global read "_Global Configuration.vi" "Resolution 12"() -> (w503:dbl[][])
                          }
                        }
                      }
                      frame True {
                        n246 = call "_Remote Communicate.vi"("DC Param"=w507, "Command"=_RT_Command."Get Table") -> ("error out"=w504:errorcluster, "Info"=w508:string)  [unwired: 4 in, 2 out]
                        n247 = Unflatten From String(type=dbl[][] [] ("Cal-"), binary string=w508) -> (value=w505:dbl[][])  [unwired: 1 in, 4 out]
                      }
                    }
                    n248 = case shown="4" w465 {
                      tunnel: w468 -> [w470 w471 w472 w473 w474 w475 w476 w477 w478 w479 w480 w481 w482 w483 w484 w485]
                      frame 0, Default {
                        n249 = global write "_Global Configuration.vi" "Calibration"(w470) -> ()
                      }
                      frame 1 {
                        n250 = global write "_Global Configuration.vi" "Calibration 2"(w471) -> ()
                      }
                      frame 2 {
                        n251 = global write "_Global Configuration.vi" "Calibration 3"(w472) -> ()
                      }
                      frame 3 {
                        n252 = global write "_Global Configuration.vi" "Calibration 4"(w473) -> ()
                      }
                      frame 4 {
                        n253 = global write "_Global Configuration.vi" "Resolution"(w474) -> ()
                      }
                      frame 5 {
                        n254 = global write "_Global Configuration.vi" "Resolution 2"(w475) -> ()
                      }
                      frame 6 {
                        n255 = global write "_Global Configuration.vi" "Resolution 3"(w476) -> ()
                      }
                      frame 7 {
                        n256 = global write "_Global Configuration.vi" "Resolution 4"(w477) -> ()
                      }
                      frame 8 {
                        n257 = global write "_Global Configuration.vi" "Resolution 5"(w478) -> ()
                      }
                      frame 9 {
                        n258 = global write "_Global Configuration.vi" "Resolution 6"(w479) -> ()
                      }
                      frame 10 {
                        n259 = global write "_Global Configuration.vi" "Resolution 7"(w480) -> ()
                      }
                      frame 11 {
                        n260 = global write "_Global Configuration.vi" "Resolution 8"(w481) -> ()
                      }
                      frame 12 {
                        n261 = global write "_Global Configuration.vi" "Resolution 9"(w482) -> ()
                      }
                      frame 13 {
                        n262 = global write "_Global Configuration.vi" "Resolution 10"(w483) -> ()
                      }
                      frame 14 {
                        n263 = global write "_Global Configuration.vi" "Resolution 11"(w484) -> ()
                      }
                      frame 15 {
                        n264 = global write "_Global Configuration.vi" "Resolution 12"(w485) -> ()
                      }
                    }
                    n265 = call "_Write XML Table.vi"("error in"=w469, "Table Type"=w465, "Table (2D-DBL)"=w468) -> ("error out"=w463:errorcluster, "XML String"=w466:string)  [unwired: 3 out]
                  }
                  frame "Set Table" {
                    n266 = Unbundle By Name(w511) -> ("LockServer"=w510:bool)
                    n267 = call "_Check Server Lock.vi"("LockServer"=w510, "Message In"=w515) -> ("error out"=w512:errorcluster, "Message Out"=w514:string, "Proceed"=w513:bool)  [unwired: 3 out]
                    n268 = case shown="True" w513 {
                      tunnel: [w517 w519] -> w516
                      tunnel: w514 -> [_ w518]
                      tunnel: w512 -> [w517 _]
                      frame False {
                      }
                      frame True {
                        # "Expect 2 2D-DBL table in XML format\n- 1st column is mass in amu\n- 2nd column is DAC value"
                        n269 = call "_Read XML Table.vi"("XML String"=w518) -> ("error out"=w522:errorcluster, "Table Type"=w521:i32, "Table (2D-DBL)"=w520:dbl[][])  [unwired: 1 in, 3 out]
                        n270 = case shown="0, Default" w521 {
                          tunnel: w520 -> [w524 w525 w526 w527 w528 w529 w530 w531 w532 w533 w534 w535 w536 w537 w538 w539]
                          frame 0, Default {
                            n271 = global write "_Global Configuration.vi" "Calibration"(w524) -> ()
                          }
                          frame 1 {
                            n272 = global write "_Global Configuration.vi" "Calibration 2"(w525) -> ()
                          }
                          frame 2 {
                            n273 = global write "_Global Configuration.vi" "Calibration 3"(w526) -> ()
                          }
                          frame 3 {
                            n274 = global write "_Global Configuration.vi" "Calibration 4"(w527) -> ()
                          }
                          frame 4 {
                            n275 = global write "_Global Configuration.vi" "Resolution"(w528) -> ()
                          }
                          frame 5 {
                            n276 = global write "_Global Configuration.vi" "Resolution 2"(w529) -> ()
                          }
                          frame 6 {
                            n277 = global write "_Global Configuration.vi" "Resolution 3"(w530) -> ()
                          }
                          frame 7 {
                            n278 = global write "_Global Configuration.vi" "Resolution 4"(w531) -> ()
                          }
                          frame 8 {
                            n279 = global write "_Global Configuration.vi" "Resolution 5"(w532) -> ()
                          }
                          frame 9 {
                            n280 = global write "_Global Configuration.vi" "Resolution 6"(w533) -> ()
                          }
                          frame 10 {
                            n281 = global write "_Global Configuration.vi" "Resolution 7"(w534) -> ()
                          }
                          frame 11 {
                            n282 = global write "_Global Configuration.vi" "Resolution 8"(w535) -> ()
                          }
                          frame 12 {
                            n283 = global write "_Global Configuration.vi" "Resolution 9"(w536) -> ()
                          }
                          frame 13 {
                            n284 = global write "_Global Configuration.vi" "Resolution 10"(w537) -> ()
                          }
                          frame 14 {
                            n285 = global write "_Global Configuration.vi" "Resolution 11"(w538) -> ()
                          }
                          frame 15 {
                            n286 = global write "_Global Configuration.vi" "Resolution 12"(w539) -> ()
                          }
                        }
                        n287 = call "_Remote Communicate.vi"("error in (no error)"=w522, "DC Param"=w521, "Command"=_RT_Command."Update Table") -> ("error out"=w519:errorcluster)  [unwired: 3 in, 3 out]
                      }
                    }
                  }
                  frame "Get Configuration" {
                    # "Outputs a configuration table in XML format"
                    n288 = global read "_Global Configuration.vi" "Configuration 2"() -> (w550:T15)
                    n289 = case shown="True" w551 {
                      tunnel: [_ w562] -> w541
                      tunnel: [w559 w561] -> w544
                      tunnel: w550 -> [w559 w560]
                      frame False {
                      }
                      frame True {
                        n290 = call "_Remote Communicate.vi"("Command"=_RT_Command."Get Config") -> ("error out"=w562:errorcluster, "Info"=w563:string)  [unwired: 5 in, 2 out]
                        n291 = Unflatten From String(type=w560, binary string=w563) -> (value=w561:T15)  [unwired: 1 in, 4 out]
                      }
                    }
                    n292 = Unbundle By Name(w544) -> ("Table"=w547:T16[])
                    n293 = Unbundle By Name(w541) -> ("status"=w546:bool)
                    n294 = Array Size(array=w547) -> (size(s)=w548:i32)
                    n295 = Equal To 0?(x=w548) -> (x = 0?=w549:bool)
                    n296 = Or(x=w549, y=w546) -> (x .or. y?=w545:bool)
                    n297 = case shown="False" w545 {
                      tunnel: w544 -> [w554 _]
                      tunnel: [w553 w557] -> w543
                      tunnel: [w552 _] -> w542
                      tunnel: w541 -> [_ w558]
                      frame False {
                        n298 = global write "_Global Configuration.vi" "Configuration 2"(w554) -> ()
                        n299 = call "_Write XML Configuration.vi"("Configuration"=w554) -> ("error out"=w553:errorcluster, "XML String"=w552:string)  [unwired: 1 in, 4 out]
                      }
                      frame True {
                        n300 = call "_Construct Error Cluster.vi"("error in"=w558, "reason"="8014: Failed to read configuration table from firmware.", "errorCode"=8014) -> ("error out"=w557:errorcluster)  [unwired: 1 in, 3 out]
                      }
                    }
                  }
                  frame "Reserved" {
                    # "Expects a configuration table in XML format"
                  }
                  frame "Get Memory Map" {
                    # "Outputs a list of FPGA memory slot mapping in text format"
                    n301 = call "_Remote Communicate.vi"("Command"=_RT_Command."Get Param") -> ("error out"=w576:errorcluster, "Info"=w566:string)  [unwired: 5 in, 2 out]
                    n302 = Current VI's Path() -> (path=w572:path)
                    n303 = Strip Path(path=w572) -> (stripped path=w573:path)  [unwired: 1 out]
                    n304 = Strip Path(path=w573) -> (stripped path=w574:path)  [unwired: 1 out]
                    n305 = Build Path(base path=w574, name or relative path="FPGA Map.txt") -> (appended path=w567:path)
                    n306 = Write to Text File(file (use dialog)=w567, text=w566) -> (refnum out=w569:refnum<file>, error out=w568:errorcluster)  [unwired: 2 in, 1 out]
                    n307 = Close File(refnum=w569, error in=w568) -> ()  [unwired: 2 out]
                  }
                  frame "Read ADC" {
                    # "Outputs I32-integers text\nformat separated by tab"
                    n308 = call "_Remote Communicate.vi"("Command"=_RT_Command."Get Status") -> ("error out"=w591:errorcluster, "Info"=w580:string)  [unwired: 5 in, 2 out]
                    n309 = local read "Busy"() -> (w586:bool)
                    n310 = call "_Remote Communicate.vi"("error in (no error)"=w591, "Command"=_RT_Command."Get Info") -> ("error out"=w590:errorcluster, "Info"=w581:string)  [unwired: 4 in, 2 out]
                    n311 = Select(t="1", s=w586, f="0") -> (s? t:f=w579:string)
                    n312 = call "_Remote Communicate.vi"("error in (no error)"=w590, "Command"=_RT_Command."Read ADC") -> ("error out"=w594:errorcluster, "Data Array"=w588:i32[])  [unwired: 4 in, 2 out]
                    n313 = Array To Spreadsheet String(array=w588, 3:"%d" ("format string")) -> (spreadsheet string=w582:string)  [unwired: 1 out]
                    n314 = Format Into String(format string="<Status>\n<IonicaServer>\n%s\n</IonicaServer>\n<SystemStatus>\n%s\n</SystemStatus>\n<Versions>\n%s\n</Versions>\n<ADC>\n%s\n</ADC>\n</Status>", w579, w580, w581, w582) -> (resulting string=w583:string)  [unwired: 2 in, 1 out]
                  }
                  frame "Set Oscillator" {
                    # "Expects 3 U32-integers separated by space:\n- Register 0,1,6,7\n- Frequency Tunning Word (Register 2,3,4,5)\n- Chip Select (0 for Q1-FREQ, 1 for Q3-FREQ)"
                    n315 = Unbundle By Name(w597) -> ("RT Ready"=w595:bool, "LockServer"=w596:bool)
                    n316 = call "_Check Server Lock.vi"("LockServer"=w596, "Message In"=w601) -> ("error out"=w598:errorcluster, "Message Out"=w600:string, "Proceed"=w599:bool)  [unwired: 3 out]
                    n317 = case shown="True" w599 {
                      tunnel: [w604 w610] -> w603
                      tunnel: w595 -> [_ w609]
                      tunnel: w602 -> [_ w607]
                      tunnel: w600 -> [_ w605]
                      tunnel: w598 -> [w604 _]
                      frame False {
                      }
                      frame True {
                        n318 = Not(x=w609) -> (.not. x?=w608:bool)
                        n319 = Or(x=w608, y=w607) -> (x .or. y?=w606:bool)
                        n320 = case shown="False" w606 {
                          tunnel: [w617 w623] -> w610
                          tunnel: w605 -> [w611 _]
                          frame False {
                            w614 = u32 0 ("default value 1")
                            n321 = Scan From String(format string="%d %d %d", input string=w611, default 1=w614, default 2=w614, default 3=w614) -> (output 1=w615:u32, output 2=w613:u32, output 3=w612:u32)  [unwired: 2 in, 3 out]
                            n322 = Build Array(w615, w613, w612) -> (w620:u32[])
                            n323 = Flatten To String(anything=w620) -> (data string=w619:string)  [unwired: 1 in, 4 out]
                            n324 = call "_Remote Communicate.vi"("String"=w619, "Command"=_RT_Command."Set Oscillator") -> ("error out"=w617:errorcluster)  [unwired: 4 in, 3 out]
                          }
                          frame True {
                            n325 = call "_Construct Error Cluster.vi"("reason"="8016: A run is in progress or system is not ready.", "errorCode"=8016) -> ("error out"=w623:errorcluster)  [unwired: 2 in, 3 out]
                          }
                        }
                      }
                    }
                  }
                  frame "Reboot" {
                    n326 = Unbundle By Name(w625) -> ("LockServer"=w624:bool)
                    n327 = call "_Check Server Lock.vi"("LockServer"=w624, "Message In"=w627) -> ("Proceed"=w626:bool)  [unwired: 5 out]
                    n328 = case shown="True" w626 {
                      tunnel: w629 -> [_ w631]
                      tunnel: [_ w630] -> w628
                      frame False {
                      }
                      frame True {
                        n329 = stacked-sequence {
                          tunnel: w631 -> [_ w634 _]
                          tunnel: [_ w633 _] -> w630
                          frame #0 {
                            n330 = local write "Busy"(TRUE ("Busy")) -> ()
                          }
                          frame #1 {
                            n331 = case shown="True" w634 {
                              tunnel: [_ w636] -> w633
                              frame False {
                                n332 = Wait (ms)(milliseconds to wait=u32 8000) -> ()  [unwired: 1 out]
                              }
                              frame True {
                                n333 = call "_Open Preference File.vi"() -> ("error"=w638:errorcluster, "refnum"=w639:T10)  [unwired: 3 in, 3 out]
                                n334 = call-poly <vilib>:"Read Key.vi"("section"="Lens", "error in (no error)"=w638, "default value"="172.16.0.2", "key"="IPAddress" ("section"), "refnum"=w639) -> ("error out"=w644:errorcluster, "value"=w636:string, "refnum out"=w643:T10)  [unwired: 1 in, 3 out]
                                n335 = call <vilib>:"Close Config Data.vi"("error in (no error)"=w644, "write file if changed (T)"=FALSE ("write configuration file? (T)"), "refnum"=w643) -> ()  [unwired: 9 out]
                                n336 = call "_Remote Reboot.vi"("IP Address"=w636) -> ()  [unwired: 2 out]
                              }
                            }
                          }
                          frame #2 {
                            n337 = local write "Busy"(FALSE ("Busy")) -> ()
                          }
                        }
                      }
                    }
                  }
                  frame "Backup Firmware" {
                    # "Expects a valide path string"
                    n338 = Unbundle By Name(w647) -> ("LockServer"=w646:bool)
                    n339 = call "_Check Server Lock.vi"("LockServer"=w646, "Message In"=w651) -> ("error out"=w648:errorcluster, "Message Out"=w650:string, "Proceed"=w649:bool)  [unwired: 3 out]
                    n340 = case shown="True" w649 {
                      tunnel: w654 -> [_ w659]
                      tunnel: [w655 w658] -> w653
                      tunnel: w652 -> [_ w657]
                      tunnel: w650 -> [_ w656]
                      tunnel: w648 -> [w655 _]
                      frame False {
                      }
                      frame True {
                        n341 = case shown="False" w659 {
                          tunnel: [w662 w696] -> w658
                          tunnel: w656 -> [w661 _]
                          tunnel: w657 -> [w660 _]
                          frame False {
                            n342 = stacked-sequence {
                              seq-local: [_ w664 _] -> [_ _ w686]
                              tunnel: [_ _ w687] -> w662
                              tunnel: w661 -> [_ w665 _]
                              tunnel: w660 -> [_ w666 _]
                              frame #0 {
                                n343 = local write "Busy"(TRUE ("Busy")) -> ()
                              }
                              frame #1 {
                                n344 = case shown="True" w666 {
                                tunnel: [_ w675] -> w664
                                tunnel: w665 -> [_ w676]
                                frame False {
                                n345 = Wait (ms)(milliseconds to wait=u32 800) -> ()  [unwired: 1 out]
                                }
                                frame True {
                                w670 = ""
                                n346 = call "_Open Preference File.vi"() -> ("error"=w678:errorcluster, "refnum"=w679:T10)  [unwired: 3 in, 3 out]
                                n347 = String To Path(string=w676) -> (path=w671:path)
                                n348 = call-poly <vilib>:"Read Key.vi"("section"="Lens", "error in (no error)"=w678, "default value"="172.16.0.2", "key"="IPAddress" ("section"), "refnum"=w679) -> ("error out"=w684:errorcluster, "value"=w672:string, "refnum out"=w683:T10)  [unwired: 1 in, 3 out]
                                n349 = call <vilib>:"Close Config Data.vi"("error in (no error)"=w684, "write file if changed (T)"=FALSE ("write configuration file? (T)"), "refnum"=w683) -> ()  [unwired: 9 out]
                                n350 = Bundle("value"=w672, w670, w671, "Source"=enum32{"RT Target", "Folder"}."RT Target") -> (w674:T17)  [unwired: 1 out]
                                n351 = Bundle("value"=w672, w670, w671, "Source"=enum32{"RT Target", "Folder"}."Folder") -> (w673:T17)  [unwired: 1 out]
                                n352 = call "_Remote RT Copy.vi"("Image Destination"=w673, "Image Source"=w674) -> ("Error Out"=w675:errorcluster)  [unwired: 2 in, 5 out]
                                }
                                }
                              }
                              frame #2 {
                                n353 = case shown="Error" w686 {
                                selector: w686 -> [_ w691]
                                tunnel: [_ w692] -> w687
                                frame No Error {
                                }
                                frame Error {
                                n354 = Unbundle By Name(w691) -> ("source"=w689:string)
                                n355 = Concatenate Strings("8017: Failed to backup firmware due to:\n", w689) -> (w688:string)
                                n356 = call "_Construct Error Cluster.vi"("reason"=w688, "errorCode"=8017) -> ("error out"=w692:errorcluster)  [unwired: 2 in, 3 out]
                                }
                                }
                                n357 = local write "Busy"(FALSE ("Busy")) -> ()
                              }
                            }
                          }
                          frame True {
                            n358 = call "_Construct Error Cluster.vi"("reason"="8016: A run is in progress or system is not ready.", "errorCode"=8016) -> ("error out"=w696:errorcluster)  [unwired: 2 in, 3 out]
                          }
                        }
                      }
                    }
                  }
                  frame "Update Firmware" {
                    # "Expects a valide path string"
                    n359 = Unbundle By Name(w698) -> ("LockServer"=w697:bool)
                    n360 = call "_Check Server Lock.vi"("LockServer"=w697, "Message In"=w702) -> ("error out"=w699:errorcluster, "Message Out"=w701:string, "Proceed"=w700:bool)  [unwired: 3 out]
                    n361 = case shown="True" w700 {
                      tunnel: w705 -> [_ w710]
                      tunnel: [w706 w709] -> w704
                      tunnel: w703 -> [_ w708]
                      tunnel: w701 -> [_ w707]
                      tunnel: w699 -> [w706 _]
                      frame False {
                      }
                      frame True {
                        n362 = case shown="False" w710 {
                          tunnel: [w713 w748] -> w709
                          tunnel: w707 -> [w712 _]
                          tunnel: w708 -> [w711 _]
                          frame False {
                            n363 = stacked-sequence {
                              seq-local: [_ w715 _] -> [_ _ w741]
                              tunnel: [_ _ w740] -> w713
                              tunnel: w712 -> [_ w717 _]
                              tunnel: w711 -> [_ w716 _]
                              frame #0 {
                                n364 = local write "Busy"(TRUE ("Busy")) -> ()
                              }
                              frame #1 {
                                n365 = case shown="True" w716 {
                                tunnel: [_ w721] -> w715
                                tunnel: w717 -> [_ w730]
                                frame False {
                                n366 = Wait (ms)(milliseconds to wait=u32 8000) -> ()  [unwired: 1 out]
                                }
                                frame True {
                                w726 = ""
                                n367 = call "_Open Preference File.vi"() -> ("error"=w732:errorcluster, "refnum"=w733:T10)  [unwired: 3 in, 3 out]
                                n368 = String To Path(string=w730) -> (path=w727:path)
                                n369 = call-poly <vilib>:"Read Key.vi"("section"="Lens", "error in (no error)"=w732, "default value"="172.16.0.2", "key"="IPAddress" ("section"), "refnum"=w733) -> ("error out"=w738:errorcluster, "value"=w720:string, "refnum out"=w737:T10)  [unwired: 1 in, 3 out]
                                n370 = call <vilib>:"Close Config Data.vi"("error in (no error)"=w738, "write file if changed (T)"=FALSE ("write configuration file? (T)"), "refnum"=w737) -> ()  [unwired: 9 out]
                                n371 = Bundle("value"=w720, w726, w727, "Source"=enum32{"RT Target", "Folder"}."Folder") -> (w729:T17)  [unwired: 1 out]
                                n372 = Bundle("value"=w720, w726, w727, "Source"=enum32{"RT Target", "Folder"}."RT Target") -> (w728:T17)  [unwired: 1 out]
                                n373 = call "_Remote RT Copy.vi"("Image Destination"=w728, "Image Source"=w729) -> ("Error Out"=w722:errorcluster)  [unwired: 2 in, 5 out]
                                n374 = call "_Remote Connect.vi"("error in (no error)"=w722, "IP Address"=w720) -> ("error out"=w723:errorcluster, "TCP"=w719:bool)  [unwired: 4 out]
                                n375 = local write "Connected"(w719) -> ()
                                n376 = call "_Load Config File.vi"("error in (no error)"=w723) -> ("error out"=w721:errorcluster)  [unwired: 6 out]
                                }
                                }
                              }
                              frame #2 {
                                n377 = case shown="Error" w741 {
                                selector: w741 -> [_ w745]
                                tunnel: [_ w746] -> w740
                                frame No Error {
                                }
                                frame Error {
                                n378 = Unbundle By Name(w745) -> ("source"=w743:string)
                                n379 = Concatenate Strings("8018: Failed to update firmware due to:\n", w743) -> (w742:string)
                                n380 = call "_Construct Error Cluster.vi"("reason"=w742, "errorCode"=8018) -> ("error out"=w746:errorcluster)  [unwired: 2 in, 3 out]
                                }
                                }
                                n381 = local write "Busy"(FALSE ("Busy")) -> ()
                              }
                            }
                          }
                          frame True {
                            n382 = call "_Construct Error Cluster.vi"("reason"="8016: A run is in progress or system is not ready.", "errorCode"=8016) -> ("error out"=w748:errorcluster)  [unwired: 2 in, 3 out]
                          }
                        }
                      }
                    }
                  }
                  frame "Auxiliary Update" {
                    n383 = Unbundle By Name(w752) -> ("LockServer"=w751:bool)
                    n384 = call "_Check Server Lock.vi"("LockServer"=w751, "Message In"=w756) -> ("error out"=w754:errorcluster, "Message Out"=w755:string, "Proceed"=w753:bool)  [unwired: 3 out]
                    n385 = case shown="True" w753 {
                      tunnel: [w759 w763] -> w758
                      tunnel: [_ w762] -> w757
                      tunnel: w755 -> [_ w761]
                      tunnel: w754 -> [w759 w760]
                      frame False {
                      }
                      frame True {
                        n386 = call "_Remote Communicate.vi"("String"=w761, "error in (no error)"=w760, "Command"=_RT_Command."Auxiliary Update") -> ("error out"=w763:errorcluster, "Info"=w762:string)  [unwired: 3 in, 2 out]
                      }
                    }
                  }
                  frame "System Status" {
                    n387 = call "_Remote Communicate.vi"("Command"=_RT_Command."Get Detail Status") -> ("error out"=w777:errorcluster, "Info"=w774:string)  [unwired: 5 in, 2 out]
                    n388 = Match Pattern(string=w774, regular expression="<Log>" ("format string")) -> (after substring=w776:string)  [unwired: 4 out]
                    n389 = Match Pattern(string=w776, regular expression="</Log>" ("format string")) -> (before substring=w770:string)  [unwired: 4 out]
                    n390 = String Subset(string=w770, offset (0)=1 ("default value 1")) -> (substring=w771:string)  [unwired: 1 out]
                    n391 = call <vilib>:"Trim Whitespace.vi"("string"=w771) -> ("trimmed string"=w765:string)  [unwired: 1 in]
                    n392 = Empty String/Path?(string/path=w765) -> (empty?=w769:bool)
                    n393 = Concatenate Strings("RT Log:\n", w765) -> (w766:string)
                    n394 = case shown="False" w769 {
                      tunnel: w766 -> [w780 _]
                      frame False {
                        n395 = call "_LogFirmwareEvents.vi"("Event"=w780) -> ()
                        n396 = call "_Log Events.vi"("Event"=w780, "Log Command"=_Log_Command."Write" ("File Command")) -> (">10MB"=w779:bool)  [unwired: 6 in, 1 out]
                        n397 = case shown="True" w779 {
                          frame False {
                          }
                          frame True {
                            n398 = call "_Log Events.vi"("Log Command"=_Log_Command."Open" ("File Command")) -> ()  [unwired: 7 in, 2 out]
                          }
                        }
                      }
                      frame True {
                      }
                    }
                  }
                  frame "Start System" {
                    n399 = Unbundle By Name(w784) -> ("LockServer"=w783:bool)
                    n400 = call "_Check Server Lock.vi"("LockServer"=w783, "Message In"=w787) -> ("error out"=w786:errorcluster, "Proceed"=w785:bool)  [unwired: 4 out]
                    n401 = case shown="True" w785 {
                      tunnel: [w789 w791] -> w788
                      tunnel: w786 -> [w789 w790]
                      frame False {
                      }
                      frame True {
                        n402 = call "_Remote Communicate.vi"("error in (no error)"=w790, "DC Param"=u16 0, "Command"=_RT_Command."Toggle Power") -> ("error out"=w791:errorcluster)  [unwired: 3 in, 3 out]
                      }
                    }
                  }
                  frame "Shutdown System" {
                    n403 = Unbundle By Name(w795) -> ("LockServer"=w794:bool)
                    n404 = call "_Check Server Lock.vi"("LockServer"=w794, "Message In"=w798) -> ("error out"=w797:errorcluster, "Proceed"=w796:bool)  [unwired: 4 out]
                    n405 = case shown="True" w796 {
                      tunnel: [w800 w802] -> w799
                      tunnel: w797 -> [w800 w801]
                      frame False {
                      }
                      frame True {
                        n406 = call "_Remote Communicate.vi"("error in (no error)"=w801, "DC Param"=u16 2, "Command"=_RT_Command."Toggle Power") -> ("error out"=w802:errorcluster)  [unwired: 3 in, 3 out]
                      }
                    }
                  }
                  frame "Set LC Input Logic" {
                    n407 = disable-structure shown="Enabled" {
                      disable-tunnel: w810 -> [w812 w815]
                      disable-tunnel: [w811 w814] -> w808
                      frame Disabled {
                        n408 = Type Cast(type=u16 0, x=w812) -> (*(type *) &x=w811:u16)
                      }
                      frame Enabled {
                        n409 = Scan From String(format string="%d", input string=w815, default 1=u16 0) -> (output 1=w814:u16)  [unwired: 2 in, 3 out]
                      }
                    }
                    n410 = call "_Remote Communicate.vi"("DC Param"=w808, "Command"=_RT_Command."Set CC Input Logics") -> ("error out"=w807:errorcluster, "Info"=w806:string)  [unwired: 4 in, 2 out]
                  }
                  frame "Set LC Hold Logic" {
                    n411 = disable-structure shown="Enabled" {
                      disable-tunnel: w819 -> [w825 w828]
                      disable-tunnel: [w824 w827] -> w818
                      frame Disabled {
                        n412 = Type Cast(type=u16 0, x=w825) -> (*(type *) &x=w824:u16)
                      }
                      frame Enabled {
                        n413 = Scan From String(format string="%d", input string=w828, default 1=u16 0) -> (output 1=w827:u16)  [unwired: 2 in, 3 out]
                      }
                    }
                    n414 = call "_Remote Communicate.vi"("DC Param"=w818, "Command"=_RT_Command."Set CC Logics") -> ("error out"=w822:errorcluster, "Info"=w821:string)  [unwired: 4 in, 2 out]
                  }
                  frame "Lock Server" {
                    n415 = Equal?(x=w838, y="1") -> (x = y?=w833:bool)
                    n416 = And(x=w836, y=w833) -> (x .and. y?=w835:bool)
                    n417 = case shown="True" w835 {
                      tunnel: [_ w843] -> w834
                      tunnel: w833 -> [w840 _]
                      tunnel: w832 -> [w841 w842]
                      tunnel: [w839 w842] -> w831
                      frame False {
                        n418 = Bundle By Name(cluster=w841, "LockServer"=w840) -> (w839:T13)
                      }
                      frame True {
                        n419 = call "_Construct Error Cluster.vi"("reason"="8028: A run is in progress and cannot be locked down for auto-tuning.", "errorCode"=8028) -> ("error out"=w843:errorcluster)  [unwired: 2 in, 3 out]
                      }
                    }
                  }
                  frame Default {
                    n420 = To Long Integer(number=w852) -> (32bit integer=w851:i32)
                    n421 = Format Into String(format string="8012: Interface command, \"%s\" or %d, is not recognized.", w852, w851) -> (resulting string=w849:string)  [unwired: 2 in, 1 out]
                    n422 = call "_Construct Error Cluster.vi"("reason"=w849, "errorCode"=8012) -> ("error out"=w848:errorcluster)  [unwired: 2 in, 3 out]
                  }
                }
                "Data" <- w235
                n423 = Unbundle By Name(w229) -> ("source"=→"Error":string)
              }
              frame #2 {
                n424 = call <vilib>:"Unset Busy.vi"() -> ()  [unwired: 11 in, 1 out]
                n425 = Format Into String(format string="Command, %s, processed: %s", w860, w855) -> (resulting string=w856:string)  [unwired: 2 in, 1 out]
                n426 = call "_Log Events.vi"("error in (no error)"=w857, "Event"=w856, "Log Command"=_Log_Command."Write" ("File Command")) -> ()  [unwired: 5 in, 2 out]
                "Ready" <- TRUE ("Ready")
              }
            }
          }
          event "GetStatus": Value Change {
            w874 = T18 3 items=["None", "ESI", "APCI", "APPI"] ("y")
            n427 = event-data() -> ()  [unwired: 2 out]
            n428 = Unbundle By Name(w868) -> ("RT Ready"=w867:bool, "InstrState"=w866:T12)
            n429 = call "_Remote Get Brief Status.vi"("For Server? (F)"=TRUE) -> ("Status"=w877:T19, "error out"=w865:errorcluster)  [unwired: 1 in, 1 out]
            n430 = local write "GetStatus"(FALSE ("GetStatus")) -> ()
            n431 = call "_Remote Get RT Status.vi"("RT Ready"=w867, "error in (no error)"=w865) -> ("InstrState"=w862:T12, "RT Ready Out"=w864:bool, "StatusIndicator"=→"MS Ready":u16)
            n432 = Not Equal?(x=w862, y=w866) -> (x != y?=w869:bool)
            n433 = case shown="True" w869 {
              tunnel: w862 -> [_ w903]
              frame False {
              }
              frame True {
                n434 = global read "_Global Configuration.vi" "TCP"() -> (w905:bool)
                n435 = Select(t="Connected", s=w905, f="Simulation") -> (s? t:f=w902:string)
                n436 = Format Into String(format string="%s (State = %s)", w902, w903) -> (resulting string=→"MS Status":string)  [unwired: 2 in, 1 out]
              }
            }
            n437 = global write "_Global Configuration.vi" "MS State"(w862) -> ()
            n438 = global write "_Server Global.vi" "MSStatus"(w877) -> ()
            n439 = Unbundle By Name(w877) -> ("Corona Discharge:"=→"Corona Discharge:":sgl, "Source 1 Voltage:"=→"ElectroSpray V1:":sgl, "Source 2 Voltage:"=→"ElectroSpray V2:":sgl, "Source 1 Type:"=w876:T18, "Source 2 Type:"=w875:T18, "Probe Temp 1:"=→"S1Temp":sgl, "Probe Temp 2:"=→"S2Temp":sgl, "HSID Temp:"=→"HSIDTemp":sgl, "Vac. Pressure:"=→"Vac. Pressure:":sgl, "Interlock OK"=→"Interlock OK":bool, "CurGas OK"=→"CurGas OK":bool, "Pump OK"=→"Pump OK":bool, "Exhaust OK"=→"Exhaust OK":bool, "Nebulizer Gas 1:"=→"Nebulizer Gas 1:":sgl, "Heating Gas 1:"=→"Heating Gas 1:":sgl, "Nebulizer Gas 2:"=→"Nebulizer Gas 2:":sgl, "Heating Gas 2:"=→"Heating Gas 2:":sgl, "Collision Gas:"=→"Collision Pressure:":sgl, "Exhaust:"=→"Exhaust:":sgl, "Dry Gas:"=→"Dry Gas:":sgl, "Pump Speed:"=→"Pump Speed:":sgl)
            "S1Type" <- w876
            "S2Type" <- w875
            n440 = Tick Count (ms)() -> (millisecond timer value=w882:u32)
            n441 = Bundle By Name(cluster=w868, "LastGetStatusTime"=w882, "InstrState"=w862, "RT Ready"=w864) -> (w881:T13)
            n442 = Equal?(x=w876, y=w874) -> (x = y?=w873:bool)
            n443 = Equal?(x=w875, y=w874) -> (x = y?=w872:bool)
            n444 = Or(x=w873, y=w872) -> (x .or. y?=w871:bool)
            n445 = Not(x=w871) -> (.not. x?=w870:bool)
            n446 = global write "_Server Global.vi" "APPI"(w871) -> ()
            n447 = property on="S1Temp" class="DigNum (strict)"("Visible"=w870) -> ()  [unwired: 2 in, 2 out]
          }
          event "ContactClosures": Value Change {
            # "Contact Closure SetUp (LC) to be removed from Ionica Server and implemented instead in Molana/Hardware Configuration/LC SetUp."
            n448 = event-data() -> ()  [unwired: 2 out]
            n449 = Unbundle By Name(w912) -> ("LockServer"=w911:bool)
            n450 = local write "ContactClosures"(FALSE ("GetStatus")) -> ()
            n451 = local read "Busy"() -> (w910:bool)
            n452 = Or(x=w911, y=w910) -> (x .or. y?=w909:bool)
            n453 = case shown="True" w909 {
              frame False {
                n454 = call "Get CC Logics.vi"() -> ()  [unwired: 8 in]
              }
              frame True {
              }
            }
          }
          event "Positive", "Negative": Value Change {
            n455 = event-data() -> ()  [unwired: 2 out]
            n456 = Unbundle By Name(w916) -> ("RT Ready"=w915:bool)
            n457 = local read "Busy"() -> (w918:bool)
            n458 = Not(x=w915) -> (.not. x?=w917:bool)
            n459 = Or(x=w917, y=w918) -> (x .or. y?=w914:bool)
            n460 = stacked-sequence {
              tunnel: w914 -> [_ w921 _]
              tunnel: "Positive" -> [_ w920 _]
              frame #0 {
                n461 = local write "Locked"(TRUE ("Locked")) -> ()
              }
              frame #1 {
                n462 = case shown="False" w921 {
                  tunnel: w920 -> [w924 _]
                  frame False {
                    w931 = T18 1 items=["None", "ESI", "APCI"] ("y")
                    # "Check for the source type"
                    n463 = global read "_Global Configuration.vi" "Single Source"() -> (w930:bool)
                    n464 = local read "S1Type"() -> (w933:i8)
                    n465 = local read "S2Type"() -> (w932:i8)
                    n466 = global read "_Global Configuration.vi" "Sim"() -> (w923:bool)
                    n467 = Equal?(x=w933, y=w931) -> (x = y?=w926:bool)
                    n468 = Equal?(x=w931, y=w932) -> (x = y?=w928:bool)
                    n469 = Not(x=w930) -> (.not. x?=w929:bool)
                    n470 = Or(x=w923, y=w926) -> (x .or. y?=w922:bool)
                    n471 = And(x=w928, y=w929) -> (x .and. y?=w925:bool)
                    n472 = Or(x=w922, y=w925) -> (x .or. y?=w927:bool)
                    n473 = case shown="True" w927 {
                      tunnel: w922 -> [_ w938]
                      tunnel: w925 -> [_ w937]
                      tunnel: w924 -> [_ w940]
                      frame False {
                        n474 = One Button Dialog(message="Cannot start auto calibration because the instrument has no ESI source." ("reason")) -> ()  [unwired: 1 in, 1 out]
                      }
                      frame True {
                        n475 = call "Update Detector Voltage.vi"("HasESI2"=w937, "HasESI1"=w938) -> ("Proceed"=w936:bool, "Run Auto-Detector Bias Procedure"=w935:bool)  [unwired: 2 in]
                        n476 = local write "Locked"(TRUE ("Locked")) -> ()
                        n477 = case shown="True" w936 {
                          tunnel: w940 -> [_ w945]
                          tunnel: w938 -> [_ w943]
                          tunnel: w937 -> [_ w942]
                          tunnel: w935 -> [_ w941]
                          frame False {
                          }
                          frame True {
                            n478 = Select(t=enum32{"Positive", "Negative"}."Positive" ("CalOption"), s=w945, f=enum32{"Positive", "Negative"}."Negative" ("CalOption")) -> (s? t:f=w944:enum32{"Positive", "Negative"})
                            n479 = call "Auto Calibration.vi"("Run Optimization Proc"=w941, "HasESI2"=w942, "HasESI1"=w943, "CalOption"=w944) -> ()  [unwired: 3 in, 1 out]
                          }
                        }
                      }
                    }
                  }
                  frame True {
                    n480 = One Button Dialog(message="Cannot start auto calibration at this time because a run is in progress or the system is not ready." ("reason")) -> ()  [unwired: 1 in, 1 out]
                  }
                }
              }
              frame #2 {
                n481 = local write "Locked"(FALSE ("Locked")) -> ()
              }
            }
          }
          event "MSStart": Value Change {
            n482 = event-data() -> ()  [unwired: 2 out]
            n483 = Unbundle By Name(w951) -> ("RT Ready"=w950:bool)
            n484 = case shown="True" w950 {
              frame False {
                n485 = call <vilib>:"Three Button Dialog.vi"("Window Title (\"\")"="Starting MS System" ("Window Title (\"\")"), "message"="Are you sure you want to start up the MS system?" ("reason")) -> ("Which Button?"=w953:T20)  [unwired: 9 in]
                n486 = Equal To 0?(x=w953) -> (x = 0?=w952:bool)
                n487 = case shown="True" w952 {
                  frame False {
                  }
                  frame True {
                    n488 = call "_Remote Communicate.vi"("DC Param"=u16 0, "Command"=_RT_Command."Toggle Power") -> ()  [unwired: 4 in, 4 out]
                  }
                }
              }
              frame True {
                # "MS system has already been started,\nno need to do anything here."
              }
            }
          }
          event "MSShutDown": Value Change {
            n489 = event-data() -> ()  [unwired: 2 out]
            n490 = call <vilib>:"Three Button Dialog.vi"("Window Title (\"\")"="Shutting down MS System" ("Window Title (\"\")"), "message"="Are you sure you want to shut down the MS system?" ("reason")) -> ("Which Button?"=w959:T20)  [unwired: 9 in]
            n491 = Equal To 0?(x=w959) -> (x = 0?=w958:bool)
            n492 = case shown="True" w958 {
              frame False {
              }
              frame True {
                # "also make sure the run is finished"
                n493 = global write "_Global Configuration.vi" "Run"(FALSE ("Running")) -> ()
                n494 = call "_Remote Communicate.vi"("DC Param"=u16 2, "Command"=_RT_Command."Toggle Power") -> ()  [unwired: 4 in, 4 out]
              }
            }
          }
          event "MSStatusWindow": Value Change {
            n495 = event-data() -> ()  [unwired: 2 out]
            n496 = disable-structure shown="Enabled" {
              disable-tunnel: [w968 TRUE ("Valid")] -> w966
              frame Disabled {
                n497 = call "Get Password.vi"("IonSniffer777"="ionics32") -> ("Valid"=w968:bool)  [unwired: 6 out]
              }
              frame Enabled {
              }
            }
            n498 = case shown="True" w966 {
              frame False {
              }
              frame True {
                n499 = vi-ref "ShowMSStatus.vi"() -> (w971:refnum<vi>)
                n500 = property class="VI"(reference=w971) -> (reference out=w972:refnum<vi>, error out=w973:errorcluster, "Front Panel.Open"=w974:bool)  [unwired: 1 in]
                n501 = case shown="True" w974 {
                  tunnel: w972 -> [w977 w983]
                  tunnel: w973 -> [w976 _]
                  tunnel: [w975 w983] -> _
                  frame False {
                    n502 = invoke class="VI" method="Run VI"(reference=w977, error in=w976, "Wait until done"=FALSE, "Auto Dispose Ref"=TRUE ("Auto Dispose Reference")) -> (reference out=w980:refnum<vi>, error out=w981:errorcluster)  [unwired: 1 in, 3 out]
                    n503 = property class="VI"(reference=w980, error in=w981, "Front Panel.Open"=TRUE ("Front Panel Window:Open")) -> (reference out=w975:refnum<vi>)  [unwired: 1 out]
                  }
                  frame True {
                  }
                }
              }
            }
          }
        }
      }
    }
    frame #3 {
      n504 = call "_Remote Communicate.vi"("DC Param"=u16 1, "Command"=_RT_Command."Ignore Error") -> ()  [unwired: 4 in, 4 out]
    }
    frame #4 {
      n505 = call "_Log Events.vi"("Log Command"=_Log_Command."Close" ("File Command")) -> ()  [unwired: 7 in, 2 out]
    }
    frame #5 {
      n506 = property class="VI"("Front Panel.Open"=FALSE ("Front Panel Window:Open")) -> ()  [unwired: 2 in, 2 out]
    }
  }
